vi "20191023_KEK_HEX5.vi"() -> ()   [LabVIEW 2017]
uses:
  <vilib>/DAQmx/create/channels.llb/DAQmx Create Channel (AI-Voltage-Basic).vi
  <vilib>/DAQmx/create/channels.llb/DAQmx Create Channel (AO-Voltage-Basic).vi
  <vilib>/DAQmx/miscellaneous.llb/DAQmx Fill In Error Info.vi
  Lake Shore Cryotronics 218.lvlib
panel:
  out "error D1":errorcluster
  out "error D2":errorcluster
  out "error U3":errorcluster
  out "error D3":errorcluster
  out "error U2":errorcluster
  out "error U1":errorcluster
  out "error S6":errorcluster
  out "error S5":errorcluster
  out "error S4":errorcluster
  out "error S3":errorcluster
  out "error S2":errorcluster
  out "error S1":errorcluster
  in  "Tab Control":T1(tab)
  out "ref LSI-D":refnum<file>
  in  "DAQ IN: P_4HeIN":tag="Dev1/ai16"
  in  "max_P4HeIN":dbl=5.0
  in  "min_P4HeIN":dbl
  in  "DAQ IN: BARA":tag="Dev1/ai7"
  in  "VISA LSI218 DOWN":refnum<visa-resource-name>="GPIB0::11::INSTR"
  in  "DAQ OUT ON?":bool
  out "ref DAQ":refnum<file>
  in  "max_OUT":dbl=5.0
  in  "min_OUT":dbl
  in  "max_FM3":dbl=5.0
  in  "min_FM3":dbl
  in  "max_FM4":dbl=5.0
  in  "min_FM4":dbl
  in  "max_dP3":dbl=5.0
  in  "min_dP3":dbl
  in  "max_dP4":dbl=5.0
  in  "min_dP4":dbl
  in  "max_LM":dbl=0.15
  in  "min_LM":dbl
  in  "max_P":dbl=5.0
  in  "min_P":dbl
  in  "DAQ IN: FM (3He)":tag="Dev1/ai6"
  in  "DAQ IN: FM (4He)":tag="Dev1/ai5"
  in  "DAQ IN: ΔP (3He)":tag="Dev1/ai4"
  in  "DAQ IN: He-level":tag="Dev1/ai2"
  in  "DAQ IN: ΔP (4He)":tag="Dev1/ai3"
  in  "DAQ IN: P (4He coil out)":tag="Dev1/ai1"
  in  "CSV filename suffix":string="TEST_"
  in  "base path":path=path "C:/Users/TUCAN_rcnp/Desktop/Labview/KEK_20191023_HEX5/TEST"
  out "ref LSI-U":refnum<file>
  in  "VISA LSI218 UP":refnum<visa-resource-name>="GPIB0::3::INSTR"
  in  "DAQ OUT":tag="Dev1/ao0"
  in  "sample #":i32=5
  out "error out \n(LSIU)":errorcluster
  out "error out\n(file creation)":errorcluster
  out "error out\n(DAQ config)":errorcluster
  out "error out\n(DAQ OUT)":errorcluster
  out "error out \n(DAQ IN)":errorcluster
  out "error out \n(record LSIU)":errorcluster
  out "error out \n(record DAQ)":errorcluster
  out "error out DAQ Final state":errorcluster
  out "error out \n(LSID)":errorcluster
  in  "max_BARA":dbl=5.0
  in  "min_BARA":dbl
  in  "min_P3HeOUT":dbl
  in  "max_P3HeOUT":dbl=5.0
  in  "DAQ IN: P_3HeOUT":tag="Dev1/ai17"
  out "error out \n(record LSID)":errorcluster
  in  "LSI-D CH":string[](array[string])=["D1", "D2", "D3", "D4", "D5", "D6", "D7", "D8"]
  in  "NI DAQ AIN labels":string[](array[string])=["P_4KRES_COILIN", "LM", "DP_3He", "DP_4He", "FM_4He", "FM_3He", "P_4KRES_BARA", "P_4He_IN", "P_3He_OUT"]
  in  "LSI-U CH labels":string[](array[string])=["U1", "U2", "U3", "U4", "U5", "U6", "U7", "U8"]
  in  "LSI-D CH labels":string[](array[string])=["D1", "D2", "D3", "DISABLED", "D5", "D6", "D7", "D8"]
  in  "LSI-U CH":string[](array[string])=["U1", "U2", "U3", "U4", "U5", "U6", "U7", "U8"]
  in  "DAQ CH":string[](array[string])=["Q1", "Q2", "Q3", "Q4", "Q5", "Q6", "Q7", "Q8", "Q9"]
  out "LSI-U Grpah 1":cluster{dbl[], dbl[]}[](graph)=[{[3644898082.6645026, 3644898087.663789, 3644898092.6640744, 3644898097.66436, 3644898102.6646466, 3644898107.663933, 3644898112.6642184, 3644898117.664504, 3644898122.66379, 3644898127.664076, 3644898132.6643624, 3644898137.665648, 3644898142.6649346, 3644898147.66522, 3644898152.6655064, 3644898157.664792, 3644898162.665078, 3644898167.665364, 3644898172.6656504, 3644898177.664936, 3644898182.665222, 3644898187.665508, 3644898192.6647944, 3644898197.66508, 3644898202.6663666, 3644898207.666652, 3644898212.6659384, 3644898217.666224, 3644898222.6665106, 3644898227.665796, 3644898232.6660824, 3644898237.667368, 3644898242.6676545, 3644898247.66694, 3644898252.6672263, 3644898257.667512, 3644898262.6667986, 3644898267.667084, 3644898272.6673694, 3644898277.667656, 3644898282.6669426, 3644898287.667228, 3644898292.6675134, 3644898297.6678, 3644898302.6680865, 3644898307.668372, 3644898312.668658, 3644898317.667944, 3644898322.6682296, 3644898327.668516, 3644898332.6678014, 3644898337.668088, 3644898342.6683736, 3644898347.66866, 3644898352.6679454, 3644898357.668232, 3644898362.6685176, 3644898367.667804, 3644898372.6680894, 3644898377.668376, 3644898382.6686616, 3644898387.667948, 3644898392.6682334, 3644898397.66852, 3644898402.6678057, 3644898407.6680913, 3644898412.6683774, 3644898417.668664, 3644898422.6679497], [305.66, 305.96, 305.22, 305.33, 305.78, 305.05, 305.43, 306.1, 305.47, 305.83, 305.61, 305.97, 305.69, 305.75, 305.82, 305.82, 305.69, 305.52, 305.52, 306.2, 306.15, 305.92, 305.78, 305.61, 305.73, 305.41, 305.57, 306.24, 306.43, 305.83, 305.97, 306.01, 306.34, 305.78, 305.78, 306.48, 306.2, 306.2, 305.47, 305.96, 305.57, 305.97, 305.83, 305.83, 306.06, 305.92, 305.66, 305.82, 305.64, 305.57, 305.78, 305.73, 306.17, 305.83, 305.9, 306.15, 305.43, 305.87, 306.24, 306.04, 305.82, 306.06, 305.52, 305.75, 306.04, 306.06, 305.48, 305.75, 305.92]}, {[3644898082.6645026, 3644898087.663789, 3644898092.6640744, 3644898097.66436, 3644898102.6646466, 3644898107.663933, 3644898112.6642184, 3644898117.664504, 3644898122.66379, 3644898127.664076, 3644898132.6643624, 3644898137.665648, 3644898142.6649346, 3644898147.66522, 3644898152.6655064, 3644898157.664792, 3644898162.665078, 3644898167.665364, 3644898172.6656504, 3644898177.664936, 3644898182.665222, 3644898187.665508, 3644898192.6647944, 3644898197.66508, 3644898202.6663666, 3644898207.666652, 3644898212.6659384, 3644898217.666224, 3644898222.6665106, 3644898227.665796, 3644898232.6660824, 3644898237.667368, 3644898242.6676545, 3644898247.66694, 3644898252.6672263, 3644898257.667512, 3644898262.6667986, 3644898267.667084, 3644898272.6673694, 3644898277.667656, 3644898282.6669426, 3644898287.667228, 3644898292.6675134, 3644898297.6678, 3644898302.6680865, 3644898307.668372, 3644898312.668658, 3644898317.667944, 3644898322.6682296, 3644898327.668516, 3644898332.6678014, 3644898337.668088, 3644898342.6683736, 3644898347.66866, 3644898352.6679454, 3644898357.668232, 3644898362.6685176, 3644898367.667804, 3644898372.6680894, 3644898377.668376, 3644898382.6686616, 3644898387.667948, 3644898392.6682334, 3644898397.66852, 3644898402.6678057, 3644898407.6680913, 3644898412.6683774, 3644898417.668664, 3644898422.6679497], [296.0, 296.1, 295.89, 295.78, 295.94, 295.91, 295.97, 296.12, 296.01, 296.1, 296.01, 296.2, 296.14, 296.06, 296.16, 296.08, 295.89, 295.97, 296.06, 296.03, 296.09, 295.99, 295.89, 295.85, 295.93, 295.74, 295.91, 296.21, 296.04, 296.14, 296.12, 295.91, 296.2, 295.91, 295.87, 296.09, 296.19, 295.91, 296.03, 296.12, 295.94, 296.03, 295.97, 296.01, 296.08, 295.89, 295.91, 295.97, 296.03, 295.81, 295.91, 296.1, 296.15, 296.05, 296.15, 296.24, 295.82, 295.81, 296.14, 296.24, 295.97, 296.06, 295.74, 295.95, 296.08, 295.94, 295.91, 295.91, 296.12]}, {[3644898082.6645026, 3644898087.663789, 3644898092.6640744, 3644898097.66436, 3644898102.6646466, 3644898107.663933, 3644898112.6642184, 3644898117.664504, 3644898122.66379, 3644898127.664076, 3644898132.6643624, 3644898137.665648, 3644898142.6649346, 3644898147.66522, 3644898152.6655064, 3644898157.664792, 3644898162.665078, 3644898167.665364, 3644898172.6656504, 3644898177.664936, 3644898182.665222, 3644898187.665508, 3644898192.6647944, 3644898197.66508, 3644898202.6663666, 3644898207.666652, 3644898212.6659384, 3644898217.666224, 3644898222.6665106, 3644898227.665796, 3644898232.6660824, 3644898237.667368, 3644898242.6676545, 3644898247.66694, 3644898252.6672263, 3644898257.667512, 3644898262.6667986, 3644898267.667084, 3644898272.6673694, 3644898277.667656, 3644898282.6669426, 3644898287.667228, 3644898292.6675134, 3644898297.6678, 3644898302.6680865, 3644898307.668372, 3644898312.668658, 3644898317.667944, 3644898322.6682296, 3644898327.668516, 3644898332.6678014, 3644898337.668088, 3644898342.6683736, 3644898347.66866, 3644898352.6679454, 3644898357.668232, 3644898362.6685176, 3644898367.667804, 3644898372.6680894, 3644898377.668376, 3644898382.6686616, 3644898387.667948, 3644898392.6682334, 3644898397.66852, 3644898402.6678057, 3644898407.6680913, 3644898412.6683774, 3644898417.668664, 3644898422.6679497], [290.48, 291.09, 290.9, 291.1, 290.9, 290.9, 291.04, 291.04, 290.99, 290.93, 290.9, 291.31, 290.97, 291.13, 291.04, 291.12, 290.93, 290.69, 291.06, 291.27, 291.06, 291.04, 290.96, 291.09, 290.86, 290.95, 291.01, 291.18, 291.25, 291.18, 290.95, 291.08, 291.12, 290.97, 290.93, 291.09, 291.27, 291.02, 290.93, 291.08, 291.22, 291.12, 290.92, 290.69, 291.02, 291.02, 290.9, 290.86, 291.08, 290.88, 290.77, 291.01, 291.05, 291.1, 291.14, 290.99, 291.06, 290.9, 291.05, 291.31, 291.05, 291.06, 290.95, 290.99, 290.99, 290.9, 290.9, 290.96, 291.08]}]
  out "LSI-U CH indic,":string[](array[string])=["U1", "U2", "U3", "U4", "U5", "U6", "U7", "U8"]
  out "LSI-U out":dbl[](array[numeric])=[305.92, 296.12, 291.08, 301.5, 302.08, 302.37, 301.36, 300.38]
  in  "GraphU1 SEL":i32[](array[numeric])=[0, 1]
  out "LSI-D out":dbl[](array[numeric])=[305.92, 296.12, 291.08, 301.5, 302.08, 302.37, 301.36, 300.38]
  out "LSI-D CH indic.":string[](array[string])=["U1", "U2", "U3", "U4", "U5", "U6", "U7", "U8"]
  out "LSI-U Grpah 2":cluster{dbl[], dbl[]}[](graph)=[{[3644898082.6645026, 3644898087.663789, 3644898092.6640744, 3644898097.66436, 3644898102.6646466, 3644898107.663933, 3644898112.6642184, 3644898117.664504, 3644898122.66379, 3644898127.664076, 3644898132.6643624, 3644898137.665648, 3644898142.6649346, 3644898147.66522, 3644898152.6655064, 3644898157.664792, 3644898162.665078, 3644898167.665364, 3644898172.6656504, 3644898177.664936, 3644898182.665222, 3644898187.665508, 3644898192.6647944, 3644898197.66508, 3644898202.6663666, 3644898207.666652, 3644898212.6659384, 3644898217.666224, 3644898222.6665106, 3644898227.665796, 3644898232.6660824, 3644898237.667368, 3644898242.6676545, 3644898247.66694, 3644898252.6672263, 3644898257.667512, 3644898262.6667986, 3644898267.667084, 3644898272.6673694, 3644898277.667656, 3644898282.6669426, 3644898287.667228, 3644898292.6675134, 3644898297.6678, 3644898302.6680865, 3644898307.668372, 3644898312.668658, 3644898317.667944, 3644898322.6682296, 3644898327.668516, 3644898332.6678014, 3644898337.668088, 3644898342.6683736, 3644898347.66866, 3644898352.6679454, 3644898357.668232, 3644898362.6685176, 3644898367.667804, 3644898372.6680894, 3644898377.668376, 3644898382.6686616, 3644898387.667948, 3644898392.6682334, 3644898397.66852, 3644898402.6678057, 3644898407.6680913, 3644898412.6683774, 3644898417.668664, 3644898422.6679497], [305.66, 305.96, 305.22, 305.33, 305.78, 305.05, 305.43, 306.1, 305.47, 305.83, 305.61, 305.97, 305.69, 305.75, 305.82, 305.82, 305.69, 305.52, 305.52, 306.2, 306.15, 305.92, 305.78, 305.61, 305.73, 305.41, 305.57, 306.24, 306.43, 305.83, 305.97, 306.01, 306.34, 305.78, 305.78, 306.48, 306.2, 306.2, 305.47, 305.96, 305.57, 305.97, 305.83, 305.83, 306.06, 305.92, 305.66, 305.82, 305.64, 305.57, 305.78, 305.73, 306.17, 305.83, 305.9, 306.15, 305.43, 305.87, 306.24, 306.04, 305.82, 306.06, 305.52, 305.75, 306.04, 306.06, 305.48, 305.75, 305.92]}, {[3644898082.6645026, 3644898087.663789, 3644898092.6640744, 3644898097.66436, 3644898102.6646466, 3644898107.663933, 3644898112.6642184, 3644898117.664504, 3644898122.66379, 3644898127.664076, 3644898132.6643624, 3644898137.665648, 3644898142.6649346, 3644898147.66522, 3644898152.6655064, 3644898157.664792, 3644898162.665078, 3644898167.665364, 3644898172.6656504, 3644898177.664936, 3644898182.665222, 3644898187.665508, 3644898192.6647944, 3644898197.66508, 3644898202.6663666, 3644898207.666652, 3644898212.6659384, 3644898217.666224, 3644898222.6665106, 3644898227.665796, 3644898232.6660824, 3644898237.667368, 3644898242.6676545, 3644898247.66694, 3644898252.6672263, 3644898257.667512, 3644898262.6667986, 3644898267.667084, 3644898272.6673694, 3644898277.667656, 3644898282.6669426, 3644898287.667228, 3644898292.6675134, 3644898297.6678, 3644898302.6680865, 3644898307.668372, 3644898312.668658, 3644898317.667944, 3644898322.6682296, 3644898327.668516, 3644898332.6678014, 3644898337.668088, 3644898342.6683736, 3644898347.66866, 3644898352.6679454, 3644898357.668232, 3644898362.6685176, 3644898367.667804, 3644898372.6680894, 3644898377.668376, 3644898382.6686616, 3644898387.667948, 3644898392.6682334, 3644898397.66852, 3644898402.6678057, 3644898407.6680913, 3644898412.6683774, 3644898417.668664, 3644898422.6679497], [296.0, 296.1, 295.89, 295.78, 295.94, 295.91, 295.97, 296.12, 296.01, 296.1, 296.01, 296.2, 296.14, 296.06, 296.16, 296.08, 295.89, 295.97, 296.06, 296.03, 296.09, 295.99, 295.89, 295.85, 295.93, 295.74, 295.91, 296.21, 296.04, 296.14, 296.12, 295.91, 296.2, 295.91, 295.87, 296.09, 296.19, 295.91, 296.03, 296.12, 295.94, 296.03, 295.97, 296.01, 296.08, 295.89, 295.91, 295.97, 296.03, 295.81, 295.91, 296.1, 296.15, 296.05, 296.15, 296.24, 295.82, 295.81, 296.14, 296.24, 295.97, 296.06, 295.74, 295.95, 296.08, 295.94, 295.91, 295.91, 296.12]}, {[3644898082.6645026, 3644898087.663789, 3644898092.6640744, 3644898097.66436, 3644898102.6646466, 3644898107.663933, 3644898112.6642184, 3644898117.664504, 3644898122.66379, 3644898127.664076, 3644898132.6643624, 3644898137.665648, 3644898142.6649346, 3644898147.66522, 3644898152.6655064, 3644898157.664792, 3644898162.665078, 3644898167.665364, 3644898172.6656504, 3644898177.664936, 3644898182.665222, 3644898187.665508, 3644898192.6647944, 3644898197.66508, 3644898202.6663666, 3644898207.666652, 3644898212.6659384, 3644898217.666224, 3644898222.6665106, 3644898227.665796, 3644898232.6660824, 3644898237.667368, 3644898242.6676545, 3644898247.66694, 3644898252.6672263, 3644898257.667512, 3644898262.6667986, 3644898267.667084, 3644898272.6673694, 3644898277.667656, 3644898282.6669426, 3644898287.667228, 3644898292.6675134, 3644898297.6678, 3644898302.6680865, 3644898307.668372, 3644898312.668658, 3644898317.667944, 3644898322.6682296, 3644898327.668516, 3644898332.6678014, 3644898337.668088, 3644898342.6683736, 3644898347.66866, 3644898352.6679454, 3644898357.668232, 3644898362.6685176, 3644898367.667804, 3644898372.6680894, 3644898377.668376, 3644898382.6686616, 3644898387.667948, 3644898392.6682334, 3644898397.66852, 3644898402.6678057, 3644898407.6680913, 3644898412.6683774, 3644898417.668664, 3644898422.6679497], [290.48, 291.09, 290.9, 291.1, 290.9, 290.9, 291.04, 291.04, 290.99, 290.93, 290.9, 291.31, 290.97, 291.13, 291.04, 291.12, 290.93, 290.69, 291.06, 291.27, 291.06, 291.04, 290.96, 291.09, 290.86, 290.95, 291.01, 291.18, 291.25, 291.18, 290.95, 291.08, 291.12, 290.97, 290.93, 291.09, 291.27, 291.02, 290.93, 291.08, 291.22, 291.12, 290.92, 290.69, 291.02, 291.02, 290.9, 290.86, 291.08, 290.88, 290.77, 291.01, 291.05, 291.1, 291.14, 290.99, 291.06, 290.9, 291.05, 291.31, 291.05, 291.06, 290.95, 290.99, 290.99, 290.9, 290.9, 290.96, 291.08]}]
  in  "GraphU2 SEL":i32[](array[numeric])=[2, 3, 4]
  in  "GraphU3 SEL":i32[](array[numeric])=[5, 6, 6]
  out "LSI-U Grpah 3":cluster{dbl[], dbl[]}[](graph)=[{[3644898082.6645026, 3644898087.663789, 3644898092.6640744, 3644898097.66436, 3644898102.6646466, 3644898107.663933, 3644898112.6642184, 3644898117.664504, 3644898122.66379, 3644898127.664076, 3644898132.6643624, 3644898137.665648, 3644898142.6649346, 3644898147.66522, 3644898152.6655064, 3644898157.664792, 3644898162.665078, 3644898167.665364, 3644898172.6656504, 3644898177.664936, 3644898182.665222, 3644898187.665508, 3644898192.6647944, 3644898197.66508, 3644898202.6663666, 3644898207.666652, 3644898212.6659384, 3644898217.666224, 3644898222.6665106, 3644898227.665796, 3644898232.6660824, 3644898237.667368, 3644898242.6676545, 3644898247.66694, 3644898252.6672263, 3644898257.667512, 3644898262.6667986, 3644898267.667084, 3644898272.6673694, 3644898277.667656, 3644898282.6669426, 3644898287.667228, 3644898292.6675134, 3644898297.6678, 3644898302.6680865, 3644898307.668372, 3644898312.668658, 3644898317.667944, 3644898322.6682296, 3644898327.668516, 3644898332.6678014, 3644898337.668088, 3644898342.6683736, 3644898347.66866, 3644898352.6679454, 3644898357.668232, 3644898362.6685176, 3644898367.667804, 3644898372.6680894, 3644898377.668376, 3644898382.6686616, 3644898387.667948, 3644898392.6682334, 3644898397.66852, 3644898402.6678057, 3644898407.6680913, 3644898412.6683774, 3644898417.668664, 3644898422.6679497], [305.66, 305.96, 305.22, 305.33, 305.78, 305.05, 305.43, 306.1, 305.47, 305.83, 305.61, 305.97, 305.69, 305.75, 305.82, 305.82, 305.69, 305.52, 305.52, 306.2, 306.15, 305.92, 305.78, 305.61, 305.73, 305.41, 305.57, 306.24, 306.43, 305.83, 305.97, 306.01, 306.34, 305.78, 305.78, 306.48, 306.2, 306.2, 305.47, 305.96, 305.57, 305.97, 305.83, 305.83, 306.06, 305.92, 305.66, 305.82, 305.64, 305.57, 305.78, 305.73, 306.17, 305.83, 305.9, 306.15, 305.43, 305.87, 306.24, 306.04, 305.82, 306.06, 305.52, 305.75, 306.04, 306.06, 305.48, 305.75, 305.92]}, {[3644898082.6645026, 3644898087.663789, 3644898092.6640744, 3644898097.66436, 3644898102.6646466, 3644898107.663933, 3644898112.6642184, 3644898117.664504, 3644898122.66379, 3644898127.664076, 3644898132.6643624, 3644898137.665648, 3644898142.6649346, 3644898147.66522, 3644898152.6655064, 3644898157.664792, 3644898162.665078, 3644898167.665364, 3644898172.6656504, 3644898177.664936, 3644898182.665222, 3644898187.665508, 3644898192.6647944, 3644898197.66508, 3644898202.6663666, 3644898207.666652, 3644898212.6659384, 3644898217.666224, 3644898222.6665106, 3644898227.665796, 3644898232.6660824, 3644898237.667368, 3644898242.6676545, 3644898247.66694, 3644898252.6672263, 3644898257.667512, 3644898262.6667986, 3644898267.667084, 3644898272.6673694, 3644898277.667656, 3644898282.6669426, 3644898287.667228, 3644898292.6675134, 3644898297.6678, 3644898302.6680865, 3644898307.668372, 3644898312.668658, 3644898317.667944, 3644898322.6682296, 3644898327.668516, 3644898332.6678014, 3644898337.668088, 3644898342.6683736, 3644898347.66866, 3644898352.6679454, 3644898357.668232, 3644898362.6685176, 3644898367.667804, 3644898372.6680894, 3644898377.668376, 3644898382.6686616, 3644898387.667948, 3644898392.6682334, 3644898397.66852, 3644898402.6678057, 3644898407.6680913, 3644898412.6683774, 3644898417.668664, 3644898422.6679497], [296.0, 296.1, 295.89, 295.78, 295.94, 295.91, 295.97, 296.12, 296.01, 296.1, 296.01, 296.2, 296.14, 296.06, 296.16, 296.08, 295.89, 295.97, 296.06, 296.03, 296.09, 295.99, 295.89, 295.85, 295.93, 295.74, 295.91, 296.21, 296.04, 296.14, 296.12, 295.91, 296.2, 295.91, 295.87, 296.09, 296.19, 295.91, 296.03, 296.12, 295.94, 296.03, 295.97, 296.01, 296.08, 295.89, 295.91, 295.97, 296.03, 295.81, 295.91, 296.1, 296.15, 296.05, 296.15, 296.24, 295.82, 295.81, 296.14, 296.24, 295.97, 296.06, 295.74, 295.95, 296.08, 295.94, 295.91, 295.91, 296.12]}, {[3644898082.6645026, 3644898087.663789, 3644898092.6640744, 3644898097.66436, 3644898102.6646466, 3644898107.663933, 3644898112.6642184, 3644898117.664504, 3644898122.66379, 3644898127.664076, 3644898132.6643624, 3644898137.665648, 3644898142.6649346, 3644898147.66522, 3644898152.6655064, 3644898157.664792, 3644898162.665078, 3644898167.665364, 3644898172.6656504, 3644898177.664936, 3644898182.665222, 3644898187.665508, 3644898192.6647944, 3644898197.66508, 3644898202.6663666, 3644898207.666652, 3644898212.6659384, 3644898217.666224, 3644898222.6665106, 3644898227.665796, 3644898232.6660824, 3644898237.667368, 3644898242.6676545, 3644898247.66694, 3644898252.6672263, 3644898257.667512, 3644898262.6667986, 3644898267.667084, 3644898272.6673694, 3644898277.667656, 3644898282.6669426, 3644898287.667228, 3644898292.6675134, 3644898297.6678, 3644898302.6680865, 3644898307.668372, 3644898312.668658, 3644898317.667944, 3644898322.6682296, 3644898327.668516, 3644898332.6678014, 3644898337.668088, 3644898342.6683736, 3644898347.66866, 3644898352.6679454, 3644898357.668232, 3644898362.6685176, 3644898367.667804, 3644898372.6680894, 3644898377.668376, 3644898382.6686616, 3644898387.667948, 3644898392.6682334, 3644898397.66852, 3644898402.6678057, 3644898407.6680913, 3644898412.6683774, 3644898417.668664, 3644898422.6679497], [290.48, 291.09, 290.9, 291.1, 290.9, 290.9, 291.04, 291.04, 290.99, 290.93, 290.9, 291.31, 290.97, 291.13, 291.04, 291.12, 290.93, 290.69, 291.06, 291.27, 291.06, 291.04, 290.96, 291.09, 290.86, 290.95, 291.01, 291.18, 291.25, 291.18, 290.95, 291.08, 291.12, 290.97, 290.93, 291.09, 291.27, 291.02, 290.93, 291.08, 291.22, 291.12, 290.92, 290.69, 291.02, 291.02, 290.9, 290.86, 291.08, 290.88, 290.77, 291.01, 291.05, 291.1, 291.14, 290.99, 291.06, 290.9, 291.05, 291.31, 291.05, 291.06, 290.95, 290.99, 290.99, 290.9, 290.9, 290.96, 291.08]}]
  out "LSI-D Grpah 2":cluster{dbl[], dbl[]}[](graph)=[{[3644898082.6645026, 3644898087.663789, 3644898092.6640744, 3644898097.66436, 3644898102.6646466, 3644898107.663933, 3644898112.6642184, 3644898117.664504, 3644898122.66379, 3644898127.664076, 3644898132.6643624, 3644898137.665648, 3644898142.6649346, 3644898147.66522, 3644898152.6655064, 3644898157.664792, 3644898162.665078, 3644898167.665364, 3644898172.6656504, 3644898177.664936, 3644898182.665222, 3644898187.665508, 3644898192.6647944, 3644898197.66508, 3644898202.6663666, 3644898207.666652, 3644898212.6659384, 3644898217.666224, 3644898222.6665106, 3644898227.665796, 3644898232.6660824, 3644898237.667368, 3644898242.6676545, 3644898247.66694, 3644898252.6672263, 3644898257.667512, 3644898262.6667986, 3644898267.667084, 3644898272.6673694, 3644898277.667656, 3644898282.6669426, 3644898287.667228, 3644898292.6675134, 3644898297.6678, 3644898302.6680865, 3644898307.668372, 3644898312.668658, 3644898317.667944, 3644898322.6682296, 3644898327.668516, 3644898332.6678014, 3644898337.668088, 3644898342.6683736, 3644898347.66866, 3644898352.6679454, 3644898357.668232, 3644898362.6685176, 3644898367.667804, 3644898372.6680894, 3644898377.668376, 3644898382.6686616, 3644898387.667948, 3644898392.6682334, 3644898397.66852, 3644898402.6678057, 3644898407.6680913, 3644898412.6683774, 3644898417.668664, 3644898422.6679497], [305.66, 305.96, 305.22, 305.33, 305.78, 305.05, 305.43, 306.1, 305.47, 305.83, 305.61, 305.97, 305.69, 305.75, 305.82, 305.82, 305.69, 305.52, 305.52, 306.2, 306.15, 305.92, 305.78, 305.61, 305.73, 305.41, 305.57, 306.24, 306.43, 305.83, 305.97, 306.01, 306.34, 305.78, 305.78, 306.48, 306.2, 306.2, 305.47, 305.96, 305.57, 305.97, 305.83, 305.83, 306.06, 305.92, 305.66, 305.82, 305.64, 305.57, 305.78, 305.73, 306.17, 305.83, 305.9, 306.15, 305.43, 305.87, 306.24, 306.04, 305.82, 306.06, 305.52, 305.75, 306.04, 306.06, 305.48, 305.75, 305.92]}, {[3644898082.6645026, 3644898087.663789, 3644898092.6640744, 3644898097.66436, 3644898102.6646466, 3644898107.663933, 3644898112.6642184, 3644898117.664504, 3644898122.66379, 3644898127.664076, 3644898132.6643624, 3644898137.665648, 3644898142.6649346, 3644898147.66522, 3644898152.6655064, 3644898157.664792, 3644898162.665078, 3644898167.665364, 3644898172.6656504, 3644898177.664936, 3644898182.665222, 3644898187.665508, 3644898192.6647944, 3644898197.66508, 3644898202.6663666, 3644898207.666652, 3644898212.6659384, 3644898217.666224, 3644898222.6665106, 3644898227.665796, 3644898232.6660824, 3644898237.667368, 3644898242.6676545, 3644898247.66694, 3644898252.6672263, 3644898257.667512, 3644898262.6667986, 3644898267.667084, 3644898272.6673694, 3644898277.667656, 3644898282.6669426, 3644898287.667228, 3644898292.6675134, 3644898297.6678, 3644898302.6680865, 3644898307.668372, 3644898312.668658, 3644898317.667944, 3644898322.6682296, 3644898327.668516, 3644898332.6678014, 3644898337.668088, 3644898342.6683736, 3644898347.66866, 3644898352.6679454, 3644898357.668232, 3644898362.6685176, 3644898367.667804, 3644898372.6680894, 3644898377.668376, 3644898382.6686616, 3644898387.667948, 3644898392.6682334, 3644898397.66852, 3644898402.6678057, 3644898407.6680913, 3644898412.6683774, 3644898417.668664, 3644898422.6679497], [296.0, 296.1, 295.89, 295.78, 295.94, 295.91, 295.97, 296.12, 296.01, 296.1, 296.01, 296.2, 296.14, 296.06, 296.16, 296.08, 295.89, 295.97, 296.06, 296.03, 296.09, 295.99, 295.89, 295.85, 295.93, 295.74, 295.91, 296.21, 296.04, 296.14, 296.12, 295.91, 296.2, 295.91, 295.87, 296.09, 296.19, 295.91, 296.03, 296.12, 295.94, 296.03, 295.97, 296.01, 296.08, 295.89, 295.91, 295.97, 296.03, 295.81, 295.91, 296.1, 296.15, 296.05, 296.15, 296.24, 295.82, 295.81, 296.14, 296.24, 295.97, 296.06, 295.74, 295.95, 296.08, 295.94, 295.91, 295.91, 296.12]}, {[3644898082.6645026, 3644898087.663789, 3644898092.6640744, 3644898097.66436, 3644898102.6646466, 3644898107.663933, 3644898112.6642184, 3644898117.664504, 3644898122.66379, 3644898127.664076, 3644898132.6643624, 3644898137.665648, 3644898142.6649346, 3644898147.66522, 3644898152.6655064, 3644898157.664792, 3644898162.665078, 3644898167.665364, 3644898172.6656504, 3644898177.664936, 3644898182.665222, 3644898187.665508, 3644898192.6647944, 3644898197.66508, 3644898202.6663666, 3644898207.666652, 3644898212.6659384, 3644898217.666224, 3644898222.6665106, 3644898227.665796, 3644898232.6660824, 3644898237.667368, 3644898242.6676545, 3644898247.66694, 3644898252.6672263, 3644898257.667512, 3644898262.6667986, 3644898267.667084, 3644898272.6673694, 3644898277.667656, 3644898282.6669426, 3644898287.667228, 3644898292.6675134, 3644898297.6678, 3644898302.6680865, 3644898307.668372, 3644898312.668658, 3644898317.667944, 3644898322.6682296, 3644898327.668516, 3644898332.6678014, 3644898337.668088, 3644898342.6683736, 3644898347.66866, 3644898352.6679454, 3644898357.668232, 3644898362.6685176, 3644898367.667804, 3644898372.6680894, 3644898377.668376, 3644898382.6686616, 3644898387.667948, 3644898392.6682334, 3644898397.66852, 3644898402.6678057, 3644898407.6680913, 3644898412.6683774, 3644898417.668664, 3644898422.6679497], [290.48, 291.09, 290.9, 291.1, 290.9, 290.9, 291.04, 291.04, 290.99, 290.93, 290.9, 291.31, 290.97, 291.13, 291.04, 291.12, 290.93, 290.69, 291.06, 291.27, 291.06, 291.04, 290.96, 291.09, 290.86, 290.95, 291.01, 291.18, 291.25, 291.18, 290.95, 291.08, 291.12, 290.97, 290.93, 291.09, 291.27, 291.02, 290.93, 291.08, 291.22, 291.12, 290.92, 290.69, 291.02, 291.02, 290.9, 290.86, 291.08, 290.88, 290.77, 291.01, 291.05, 291.1, 291.14, 290.99, 291.06, 290.9, 291.05, 291.31, 291.05, 291.06, 290.95, 290.99, 290.99, 290.9, 290.9, 290.96, 291.08]}]
  out "LSI-D Grpah 3":cluster{dbl[], dbl[]}[](graph)=[{[3644898082.6645026, 3644898087.663789, 3644898092.6640744, 3644898097.66436, 3644898102.6646466, 3644898107.663933, 3644898112.6642184, 3644898117.664504, 3644898122.66379, 3644898127.664076, 3644898132.6643624, 3644898137.665648, 3644898142.6649346, 3644898147.66522, 3644898152.6655064, 3644898157.664792, 3644898162.665078, 3644898167.665364, 3644898172.6656504, 3644898177.664936, 3644898182.665222, 3644898187.665508, 3644898192.6647944, 3644898197.66508, 3644898202.6663666, 3644898207.666652, 3644898212.6659384, 3644898217.666224, 3644898222.6665106, 3644898227.665796, 3644898232.6660824, 3644898237.667368, 3644898242.6676545, 3644898247.66694, 3644898252.6672263, 3644898257.667512, 3644898262.6667986, 3644898267.667084, 3644898272.6673694, 3644898277.667656, 3644898282.6669426, 3644898287.667228, 3644898292.6675134, 3644898297.6678, 3644898302.6680865, 3644898307.668372, 3644898312.668658, 3644898317.667944, 3644898322.6682296, 3644898327.668516, 3644898332.6678014, 3644898337.668088, 3644898342.6683736, 3644898347.66866, 3644898352.6679454, 3644898357.668232, 3644898362.6685176, 3644898367.667804, 3644898372.6680894, 3644898377.668376, 3644898382.6686616, 3644898387.667948, 3644898392.6682334, 3644898397.66852, 3644898402.6678057, 3644898407.6680913, 3644898412.6683774, 3644898417.668664, 3644898422.6679497], [305.66, 305.96, 305.22, 305.33, 305.78, 305.05, 305.43, 306.1, 305.47, 305.83, 305.61, 305.97, 305.69, 305.75, 305.82, 305.82, 305.69, 305.52, 305.52, 306.2, 306.15, 305.92, 305.78, 305.61, 305.73, 305.41, 305.57, 306.24, 306.43, 305.83, 305.97, 306.01, 306.34, 305.78, 305.78, 306.48, 306.2, 306.2, 305.47, 305.96, 305.57, 305.97, 305.83, 305.83, 306.06, 305.92, 305.66, 305.82, 305.64, 305.57, 305.78, 305.73, 306.17, 305.83, 305.9, 306.15, 305.43, 305.87, 306.24, 306.04, 305.82, 306.06, 305.52, 305.75, 306.04, 306.06, 305.48, 305.75, 305.92]}, {[3644898082.6645026, 3644898087.663789, 3644898092.6640744, 3644898097.66436, 3644898102.6646466, 3644898107.663933, 3644898112.6642184, 3644898117.664504, 3644898122.66379, 3644898127.664076, 3644898132.6643624, 3644898137.665648, 3644898142.6649346, 3644898147.66522, 3644898152.6655064, 3644898157.664792, 3644898162.665078, 3644898167.665364, 3644898172.6656504, 3644898177.664936, 3644898182.665222, 3644898187.665508, 3644898192.6647944, 3644898197.66508, 3644898202.6663666, 3644898207.666652, 3644898212.6659384, 3644898217.666224, 3644898222.6665106, 3644898227.665796, 3644898232.6660824, 3644898237.667368, 3644898242.6676545, 3644898247.66694, 3644898252.6672263, 3644898257.667512, 3644898262.6667986, 3644898267.667084, 3644898272.6673694, 3644898277.667656, 3644898282.6669426, 3644898287.667228, 3644898292.6675134, 3644898297.6678, 3644898302.6680865, 3644898307.668372, 3644898312.668658, 3644898317.667944, 3644898322.6682296, 3644898327.668516, 3644898332.6678014, 3644898337.668088, 3644898342.6683736, 3644898347.66866, 3644898352.6679454, 3644898357.668232, 3644898362.6685176, 3644898367.667804, 3644898372.6680894, 3644898377.668376, 3644898382.6686616, 3644898387.667948, 3644898392.6682334, 3644898397.66852, 3644898402.6678057, 3644898407.6680913, 3644898412.6683774, 3644898417.668664, 3644898422.6679497], [296.0, 296.1, 295.89, 295.78, 295.94, 295.91, 295.97, 296.12, 296.01, 296.1, 296.01, 296.2, 296.14, 296.06, 296.16, 296.08, 295.89, 295.97, 296.06, 296.03, 296.09, 295.99, 295.89, 295.85, 295.93, 295.74, 295.91, 296.21, 296.04, 296.14, 296.12, 295.91, 296.2, 295.91, 295.87, 296.09, 296.19, 295.91, 296.03, 296.12, 295.94, 296.03, 295.97, 296.01, 296.08, 295.89, 295.91, 295.97, 296.03, 295.81, 295.91, 296.1, 296.15, 296.05, 296.15, 296.24, 295.82, 295.81, 296.14, 296.24, 295.97, 296.06, 295.74, 295.95, 296.08, 295.94, 295.91, 295.91, 296.12]}, {[3644898082.6645026, 3644898087.663789, 3644898092.6640744, 3644898097.66436, 3644898102.6646466, 3644898107.663933, 3644898112.6642184, 3644898117.664504, 3644898122.66379, 3644898127.664076, 3644898132.6643624, 3644898137.665648, 3644898142.6649346, 3644898147.66522, 3644898152.6655064, 3644898157.664792, 3644898162.665078, 3644898167.665364, 3644898172.6656504, 3644898177.664936, 3644898182.665222, 3644898187.665508, 3644898192.6647944, 3644898197.66508, 3644898202.6663666, 3644898207.666652, 3644898212.6659384, 3644898217.666224, 3644898222.6665106, 3644898227.665796, 3644898232.6660824, 3644898237.667368, 3644898242.6676545, 3644898247.66694, 3644898252.6672263, 3644898257.667512, 3644898262.6667986, 3644898267.667084, 3644898272.6673694, 3644898277.667656, 3644898282.6669426, 3644898287.667228, 3644898292.6675134, 3644898297.6678, 3644898302.6680865, 3644898307.668372, 3644898312.668658, 3644898317.667944, 3644898322.6682296, 3644898327.668516, 3644898332.6678014, 3644898337.668088, 3644898342.6683736, 3644898347.66866, 3644898352.6679454, 3644898357.668232, 3644898362.6685176, 3644898367.667804, 3644898372.6680894, 3644898377.668376, 3644898382.6686616, 3644898387.667948, 3644898392.6682334, 3644898397.66852, 3644898402.6678057, 3644898407.6680913, 3644898412.6683774, 3644898417.668664, 3644898422.6679497], [290.48, 291.09, 290.9, 291.1, 290.9, 290.9, 291.04, 291.04, 290.99, 290.93, 290.9, 291.31, 290.97, 291.13, 291.04, 291.12, 290.93, 290.69, 291.06, 291.27, 291.06, 291.04, 290.96, 291.09, 290.86, 290.95, 291.01, 291.18, 291.25, 291.18, 290.95, 291.08, 291.12, 290.97, 290.93, 291.09, 291.27, 291.02, 290.93, 291.08, 291.22, 291.12, 290.92, 290.69, 291.02, 291.02, 290.9, 290.86, 291.08, 290.88, 290.77, 291.01, 291.05, 291.1, 291.14, 290.99, 291.06, 290.9, 291.05, 291.31, 291.05, 291.06, 290.95, 290.99, 290.99, 290.9, 290.9, 290.96, 291.08]}]
  in  "GraphD1 SEL":i32[](array[numeric])=[0, 1]
  out "LSI-D Grpah 1":cluster{dbl[], dbl[]}[](graph)=[{[3644898082.6645026, 3644898087.663789, 3644898092.6640744, 3644898097.66436, 3644898102.6646466, 3644898107.663933, 3644898112.6642184, 3644898117.664504, 3644898122.66379, 3644898127.664076, 3644898132.6643624, 3644898137.665648, 3644898142.6649346, 3644898147.66522, 3644898152.6655064, 3644898157.664792, 3644898162.665078, 3644898167.665364, 3644898172.6656504, 3644898177.664936, 3644898182.665222, 3644898187.665508, 3644898192.6647944, 3644898197.66508, 3644898202.6663666, 3644898207.666652, 3644898212.6659384, 3644898217.666224, 3644898222.6665106, 3644898227.665796, 3644898232.6660824, 3644898237.667368, 3644898242.6676545, 3644898247.66694, 3644898252.6672263, 3644898257.667512, 3644898262.6667986, 3644898267.667084, 3644898272.6673694, 3644898277.667656, 3644898282.6669426, 3644898287.667228, 3644898292.6675134, 3644898297.6678, 3644898302.6680865, 3644898307.668372, 3644898312.668658, 3644898317.667944, 3644898322.6682296, 3644898327.668516, 3644898332.6678014, 3644898337.668088, 3644898342.6683736, 3644898347.66866, 3644898352.6679454, 3644898357.668232, 3644898362.6685176, 3644898367.667804, 3644898372.6680894, 3644898377.668376, 3644898382.6686616, 3644898387.667948, 3644898392.6682334, 3644898397.66852, 3644898402.6678057, 3644898407.6680913, 3644898412.6683774, 3644898417.668664, 3644898422.6679497], [305.66, 305.96, 305.22, 305.33, 305.78, 305.05, 305.43, 306.1, 305.47, 305.83, 305.61, 305.97, 305.69, 305.75, 305.82, 305.82, 305.69, 305.52, 305.52, 306.2, 306.15, 305.92, 305.78, 305.61, 305.73, 305.41, 305.57, 306.24, 306.43, 305.83, 305.97, 306.01, 306.34, 305.78, 305.78, 306.48, 306.2, 306.2, 305.47, 305.96, 305.57, 305.97, 305.83, 305.83, 306.06, 305.92, 305.66, 305.82, 305.64, 305.57, 305.78, 305.73, 306.17, 305.83, 305.9, 306.15, 305.43, 305.87, 306.24, 306.04, 305.82, 306.06, 305.52, 305.75, 306.04, 306.06, 305.48, 305.75, 305.92]}, {[3644898082.6645026, 3644898087.663789, 3644898092.6640744, 3644898097.66436, 3644898102.6646466, 3644898107.663933, 3644898112.6642184, 3644898117.664504, 3644898122.66379, 3644898127.664076, 3644898132.6643624, 3644898137.665648, 3644898142.6649346, 3644898147.66522, 3644898152.6655064, 3644898157.664792, 3644898162.665078, 3644898167.665364, 3644898172.6656504, 3644898177.664936, 3644898182.665222, 3644898187.665508, 3644898192.6647944, 3644898197.66508, 3644898202.6663666, 3644898207.666652, 3644898212.6659384, 3644898217.666224, 3644898222.6665106, 3644898227.665796, 3644898232.6660824, 3644898237.667368, 3644898242.6676545, 3644898247.66694, 3644898252.6672263, 3644898257.667512, 3644898262.6667986, 3644898267.667084, 3644898272.6673694, 3644898277.667656, 3644898282.6669426, 3644898287.667228, 3644898292.6675134, 3644898297.6678, 3644898302.6680865, 3644898307.668372, 3644898312.668658, 3644898317.667944, 3644898322.6682296, 3644898327.668516, 3644898332.6678014, 3644898337.668088, 3644898342.6683736, 3644898347.66866, 3644898352.6679454, 3644898357.668232, 3644898362.6685176, 3644898367.667804, 3644898372.6680894, 3644898377.668376, 3644898382.6686616, 3644898387.667948, 3644898392.6682334, 3644898397.66852, 3644898402.6678057, 3644898407.6680913, 3644898412.6683774, 3644898417.668664, 3644898422.6679497], [296.0, 296.1, 295.89, 295.78, 295.94, 295.91, 295.97, 296.12, 296.01, 296.1, 296.01, 296.2, 296.14, 296.06, 296.16, 296.08, 295.89, 295.97, 296.06, 296.03, 296.09, 295.99, 295.89, 295.85, 295.93, 295.74, 295.91, 296.21, 296.04, 296.14, 296.12, 295.91, 296.2, 295.91, 295.87, 296.09, 296.19, 295.91, 296.03, 296.12, 295.94, 296.03, 295.97, 296.01, 296.08, 295.89, 295.91, 295.97, 296.03, 295.81, 295.91, 296.1, 296.15, 296.05, 296.15, 296.24, 295.82, 295.81, 296.14, 296.24, 295.97, 296.06, 295.74, 295.95, 296.08, 295.94, 295.91, 295.91, 296.12]}, {[3644898082.6645026, 3644898087.663789, 3644898092.6640744, 3644898097.66436, 3644898102.6646466, 3644898107.663933, 3644898112.6642184, 3644898117.664504, 3644898122.66379, 3644898127.664076, 3644898132.6643624, 3644898137.665648, 3644898142.6649346, 3644898147.66522, 3644898152.6655064, 3644898157.664792, 3644898162.665078, 3644898167.665364, 3644898172.6656504, 3644898177.664936, 3644898182.665222, 3644898187.665508, 3644898192.6647944, 3644898197.66508, 3644898202.6663666, 3644898207.666652, 3644898212.6659384, 3644898217.666224, 3644898222.6665106, 3644898227.665796, 3644898232.6660824, 3644898237.667368, 3644898242.6676545, 3644898247.66694, 3644898252.6672263, 3644898257.667512, 3644898262.6667986, 3644898267.667084, 3644898272.6673694, 3644898277.667656, 3644898282.6669426, 3644898287.667228, 3644898292.6675134, 3644898297.6678, 3644898302.6680865, 3644898307.668372, 3644898312.668658, 3644898317.667944, 3644898322.6682296, 3644898327.668516, 3644898332.6678014, 3644898337.668088, 3644898342.6683736, 3644898347.66866, 3644898352.6679454, 3644898357.668232, 3644898362.6685176, 3644898367.667804, 3644898372.6680894, 3644898377.668376, 3644898382.6686616, 3644898387.667948, 3644898392.6682334, 3644898397.66852, 3644898402.6678057, 3644898407.6680913, 3644898412.6683774, 3644898417.668664, 3644898422.6679497], [290.48, 291.09, 290.9, 291.1, 290.9, 290.9, 291.04, 291.04, 290.99, 290.93, 290.9, 291.31, 290.97, 291.13, 291.04, 291.12, 290.93, 290.69, 291.06, 291.27, 291.06, 291.04, 290.96, 291.09, 290.86, 290.95, 291.01, 291.18, 291.25, 291.18, 290.95, 291.08, 291.12, 290.97, 290.93, 291.09, 291.27, 291.02, 290.93, 291.08, 291.22, 291.12, 290.92, 290.69, 291.02, 291.02, 290.9, 290.86, 291.08, 290.88, 290.77, 291.01, 291.05, 291.1, 291.14, 290.99, 291.06, 290.9, 291.05, 291.31, 291.05, 291.06, 290.95, 290.99, 290.99, 290.9, 290.9, 290.96, 291.08]}]
  in  "GraphD2 SEL":i32[](array[numeric])=[2, 3, 4]
  in  "GraphD3 SEL":i32[](array[numeric])=[5, 6, 6]
  out "Graph S. 6":cluster{dbl[], dbl[]}[](graph)
  in  "S.6 SEL":i32[](array[numeric])=[0, 2, 3]
  in  "log/linear 6":bool
  in  "log/linear 5":bool
  in  "S.5 SEL":i32[](array[numeric])=[0, 2, 3]
  in  "log/linear 4":bool
  in  "S.4 SEL":i32[](array[numeric])=[0, 2, 3]
  in  "log/linear 3":bool
  in  "log/linear 1":bool
  in  "unit":string[](array[string])=["Pa", "%", "Pa", "Pa", "L/min", "L/min", "Pa", "Pa", "Pa"]
  out "NI DAQ OUT":dbl[](array[numeric])=[-50013.24569663551, 15.025355709698363, -250.03334959533717, -250.04156931728906, -26.29672579614668, -0.7155199244462975, 103537.91205606361, -50000.0, -50000.0] format="%#_3f"
  out "NI-DAQ CH indic.":string[](array[string])=["U1", "U2", "U3", "U4", "U5", "U6", "U7", "U8"]
  out "Graph S. 1":cluster{dbl[], dbl[]}[](graph)
  in  "S.1 SEL":i32[](array[numeric])=[0, 2]
  out "Graph S. 2":cluster{dbl[], dbl[]}[](graph)
  in  "S.2 SEL":i32[](array[numeric])=[1]
  in  "log/linear 2":bool
  out "Graph S. 3":cluster{dbl[], dbl[]}[](graph)
  in  "S.3 SEL":i32[](array[numeric])=[0, 2, 3]
  out "Graph S. 4":cluster{dbl[], dbl[]}[](graph)
  out "Graph S. 5":cluster{dbl[], dbl[]}[](graph)
  out "date/time string":string="20190702_164122_"
  out "DAQ OUT \nsample #":u32=1
  in  "DAQ OUT SET Volt":dbl[](array[numeric])=[2.0] format="%0.2f"
  out "Cycle #":i32=68
  out "current time":timestamp=timestamp(3644898422.6679497 s since 1904-01-01)
  in  "?":bool
  in  "Wait (s)":i32=5
  # "Some time needed until program stops!"
  # "Record Config"
  # "VISA address"
  # "Error states"
  # "CH4 of LSI-D broken!"
  # "NI-DAQ config"
  # "Defines # of measurements \n taken for averaging"
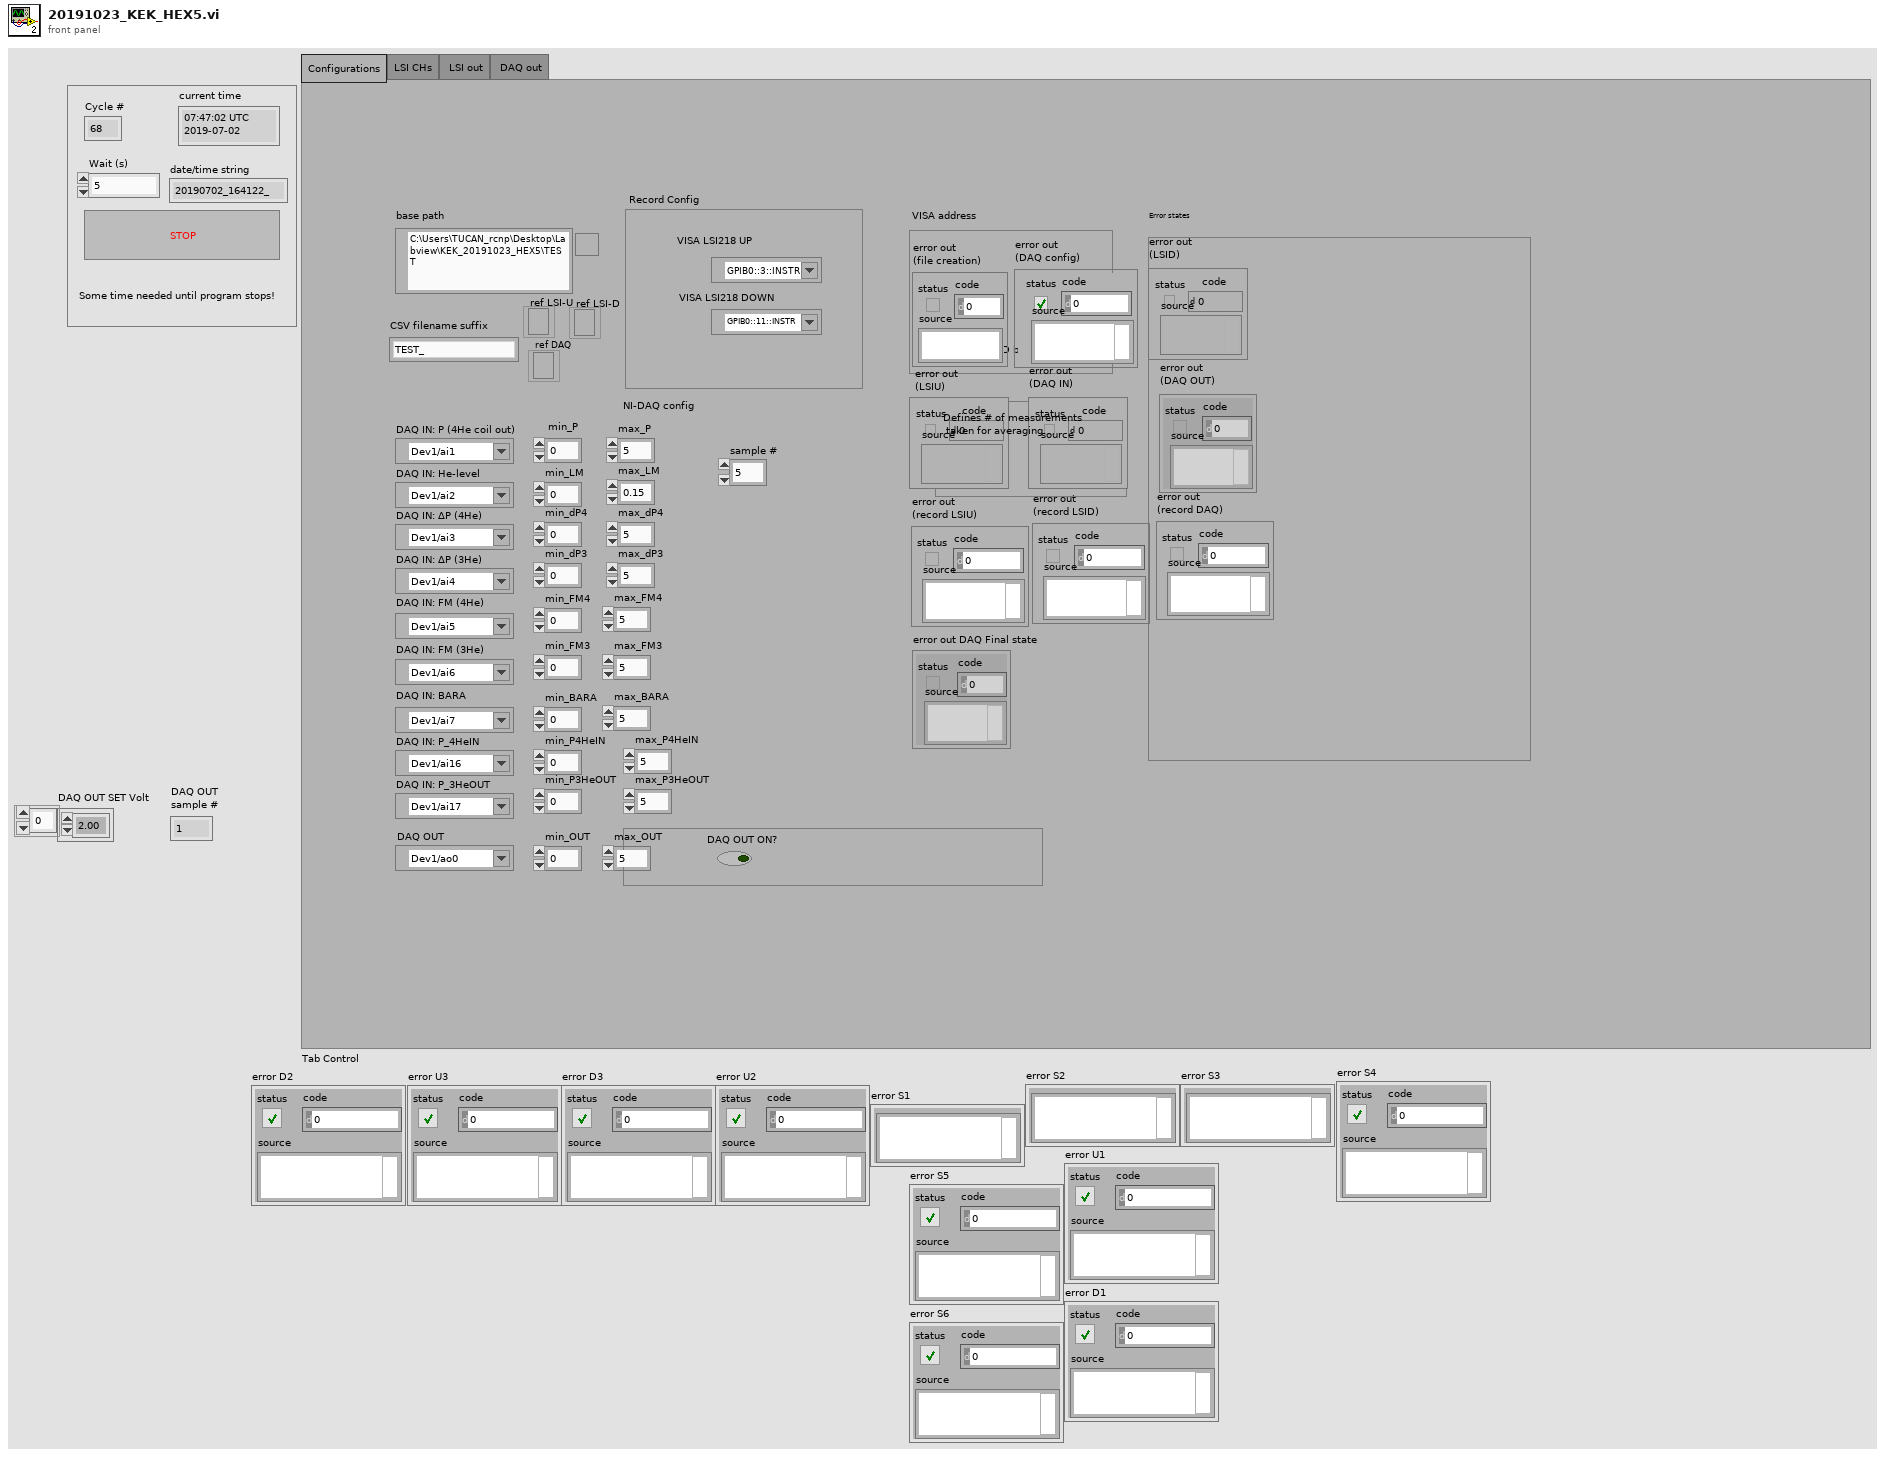
[diagram p1: front panel]
types:
  T1 = enum32{"Configurations", "LSI CHs", " LSI out", " DAQ out"}
  T2 = enum16{"open", "replace", "create", "open or create", "replace or create", "replace or create with confirmation"}
  T3 = cluster{"LSI-U CH labels[0]":string, "LSI-U CH labels[1]":string, "LSI-U CH labels[2]":string, "LSI-U CH labels[3]":string, "LSI-U CH labels[4]":string, "LSI-U CH labels[5]":string, "LSI-U CH labels[6]":string, "LSI-U CH labels[7]":string, "LSI-U CH labels[8]":string}
  T4 = cluster{"LSI-D CH labels[0]":string, "LSI-D CH labels[1]":string, "LSI-D CH labels[2]":string, "LSI-D CH labels[3]":string, "LSI-D CH labels[4]":string, "LSI-D CH labels[5]":string, "LSI-D CH labels[6]":string, "LSI-D CH labels[7]":string, "LSI-D CH labels[8]":string}
  T5 = cluster{"NI DAQ AIN labels[0]":string, "NI DAQ AIN labels[1]":string, "NI DAQ AIN labels[2]":string, "NI DAQ AIN labels[3]":string, "NI DAQ AIN labels[4]":string, "NI DAQ AIN labels[5]":string, "NI DAQ AIN labels[6]":string, "NI DAQ AIN labels[7]":string, "NI DAQ AIN labels[8]":string}
  T6 = cluster{"LSI-D out[0]":dbl, "LSI-D out[1]":dbl, "LSI-D out[2]":dbl, "LSI-D out[3]":dbl, "LSI-D out[4]":dbl, "LSI-D out[5]":dbl, "LSI-D out[6]":dbl, "LSI-D out[7]":dbl, "LSI-D out[8]":dbl}
  T7 = cluster{"LSI-U out[0]":dbl, "LSI-U out[1]":dbl, "LSI-U out[2]":dbl, "LSI-U out[3]":dbl, "LSI-U out[4]":dbl, "LSI-U out[5]":dbl, "LSI-U out[6]":dbl, "LSI-U out[7]":dbl, "LSI-U out[8]":dbl}
  T8 = cluster{"[0]":dbl, "[1]":dbl, "[2]":dbl, "[3]":dbl, "[4]":dbl, "[5]":dbl, "[6]":dbl, "[7]":dbl, "[8]":dbl}
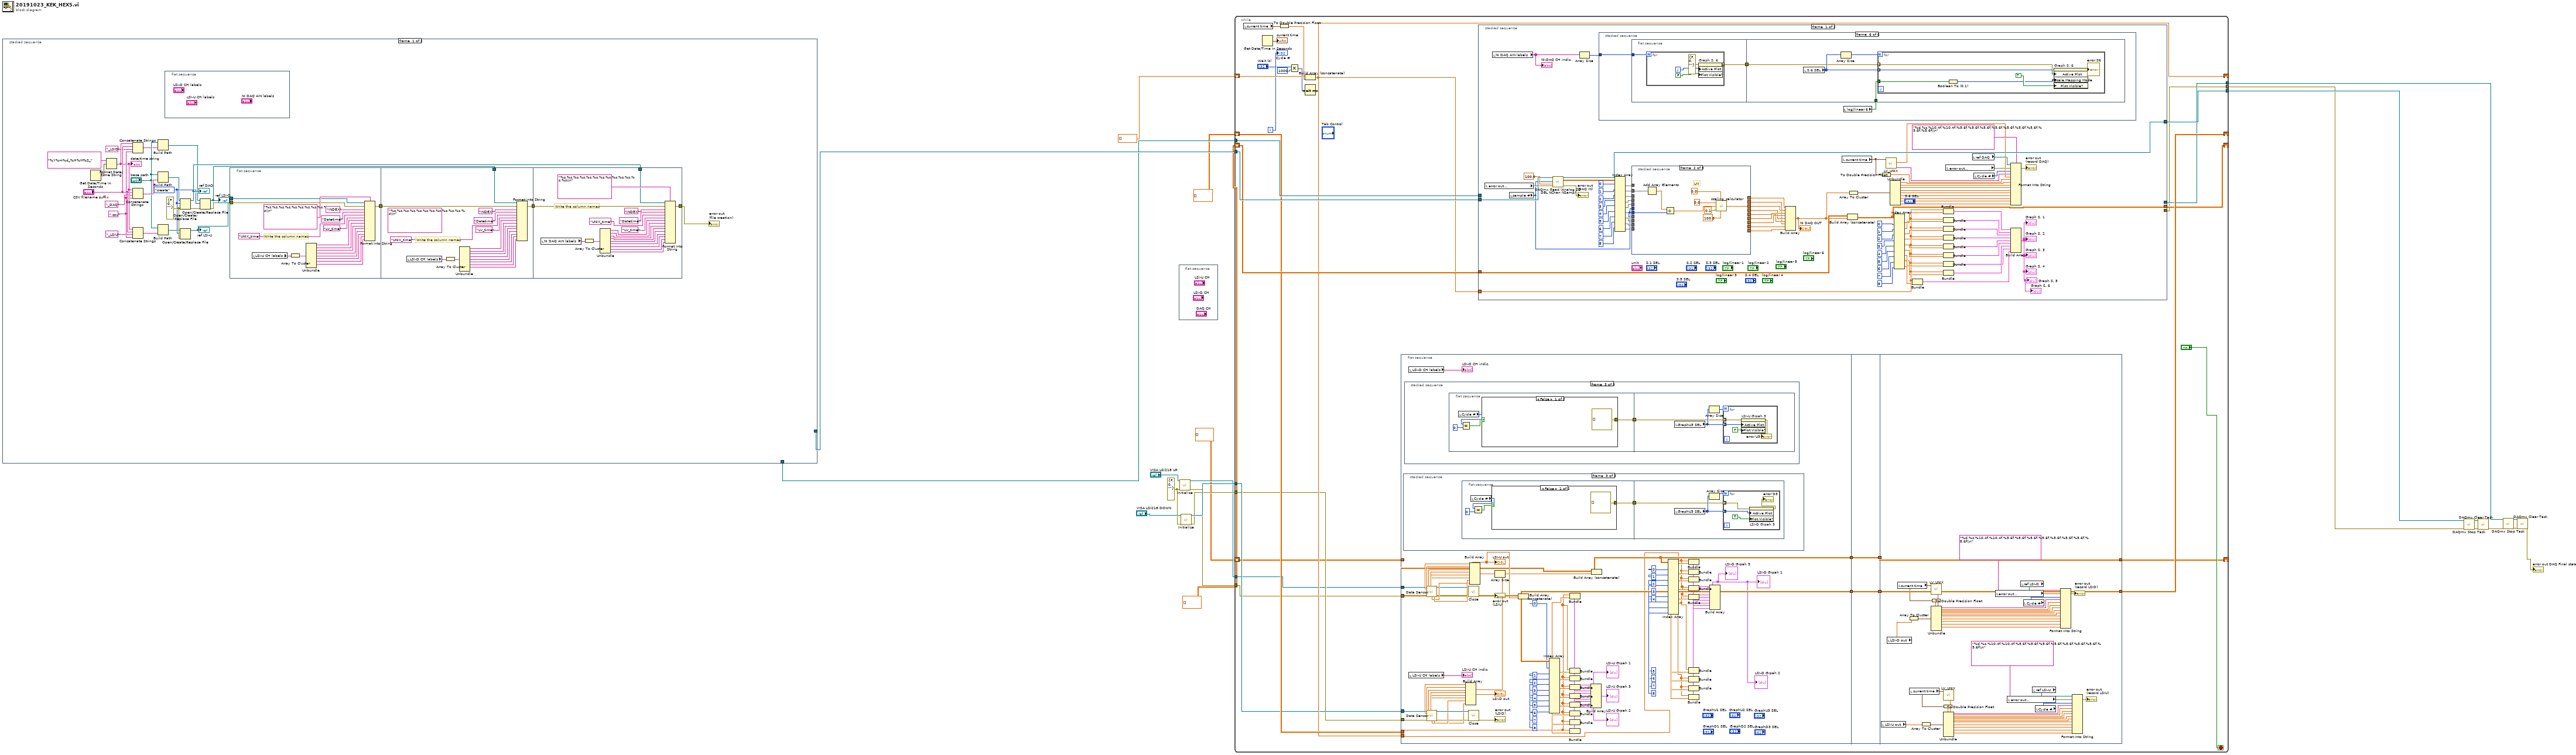
[diagram p0: block diagram]
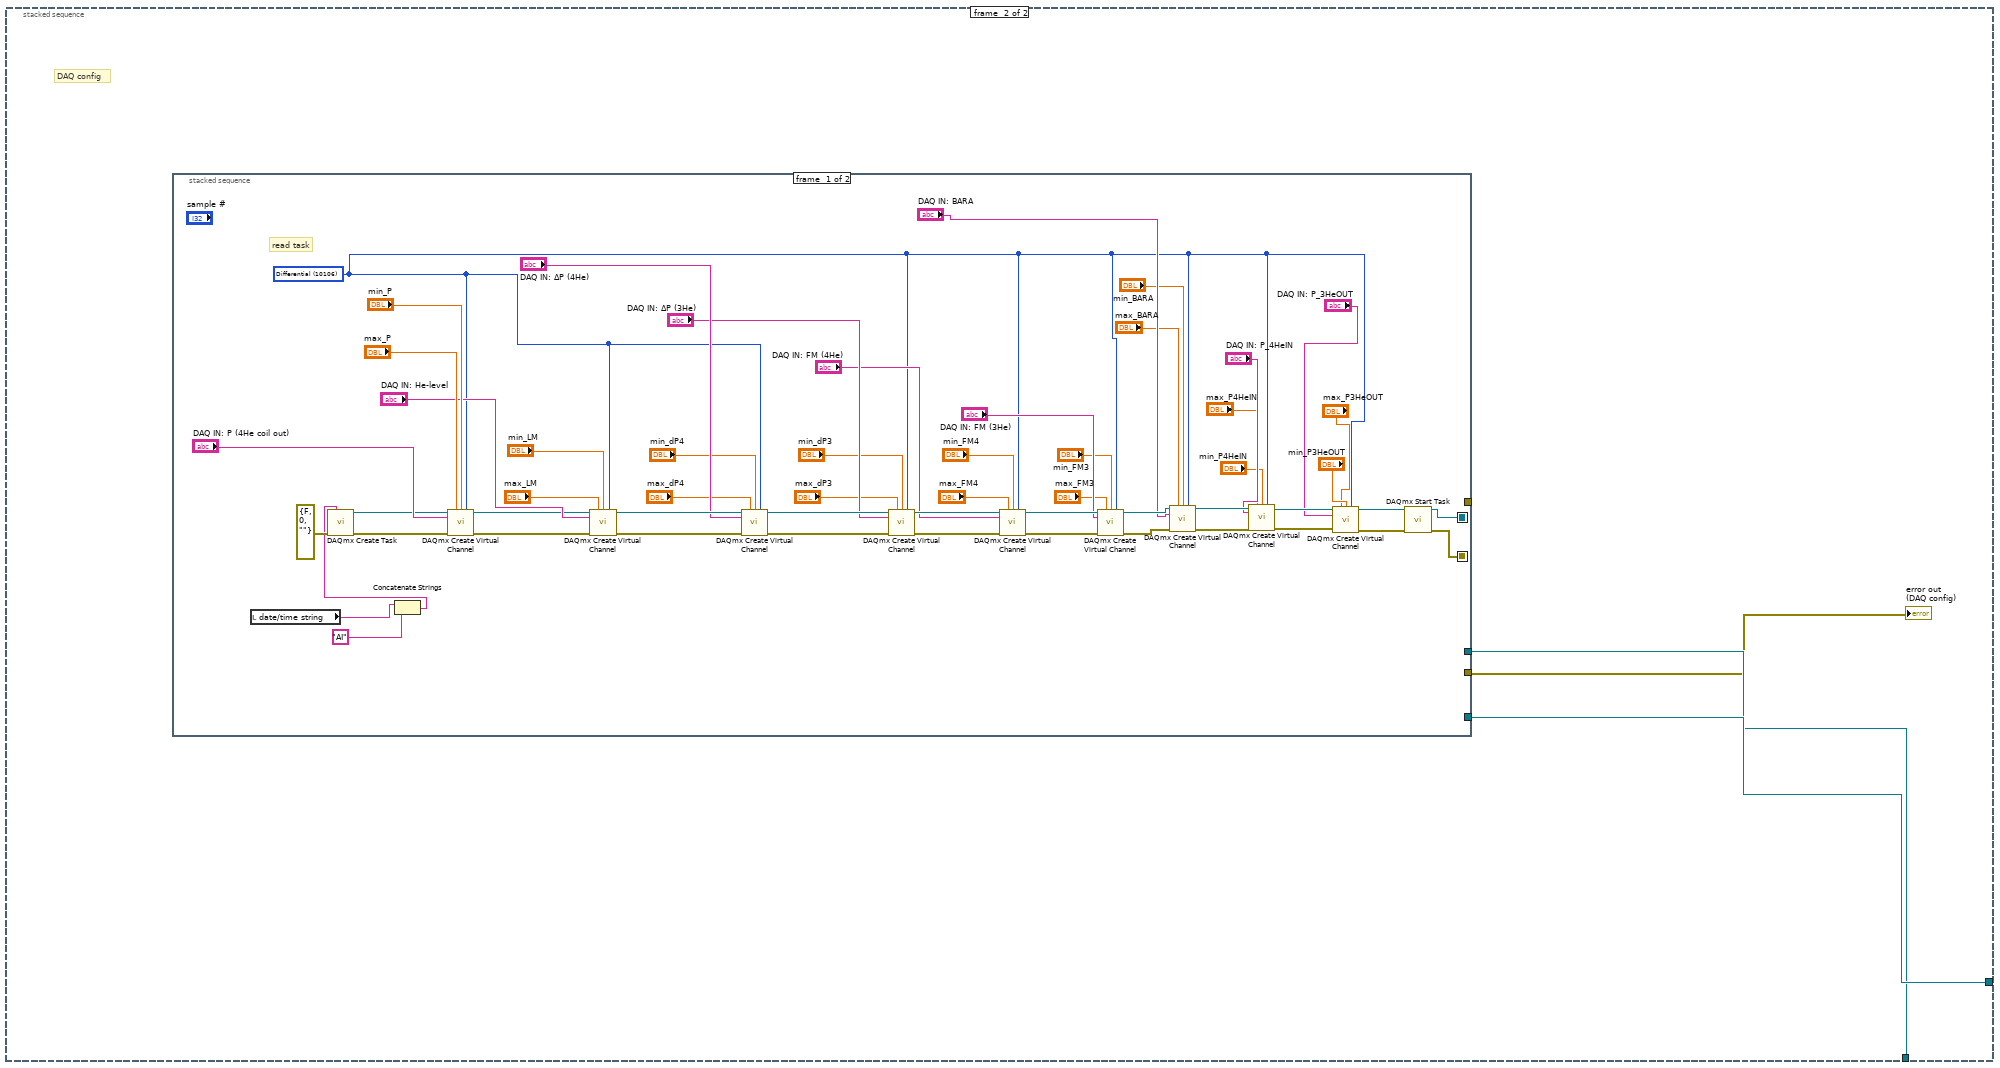
[diagram p2: hidden frame]
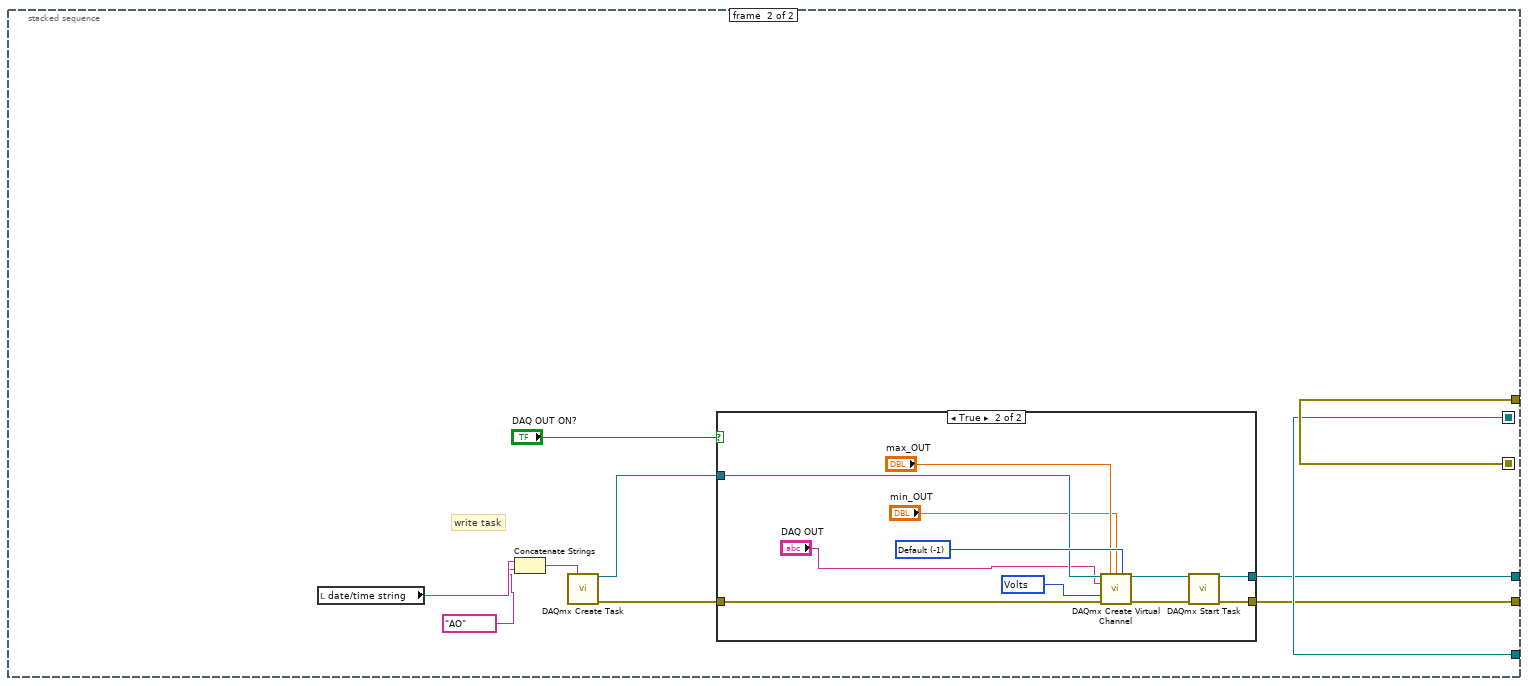
[diagram p3: hidden frame]
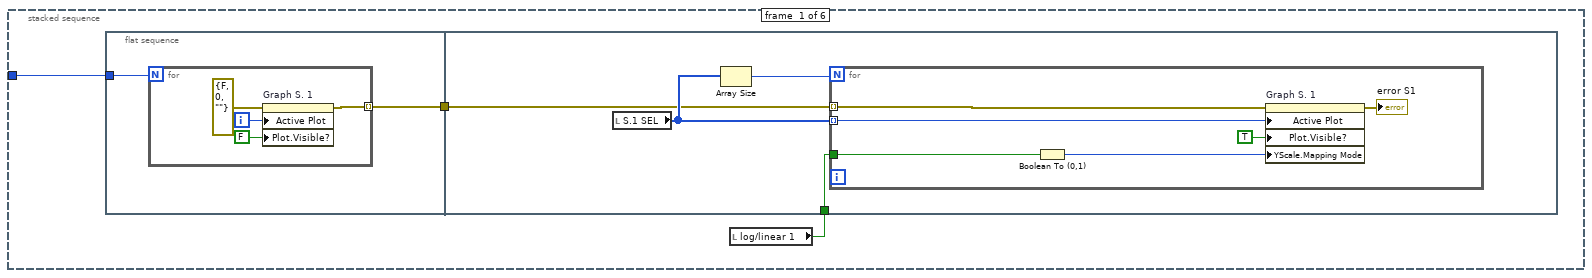
[diagram p5: hidden frame]
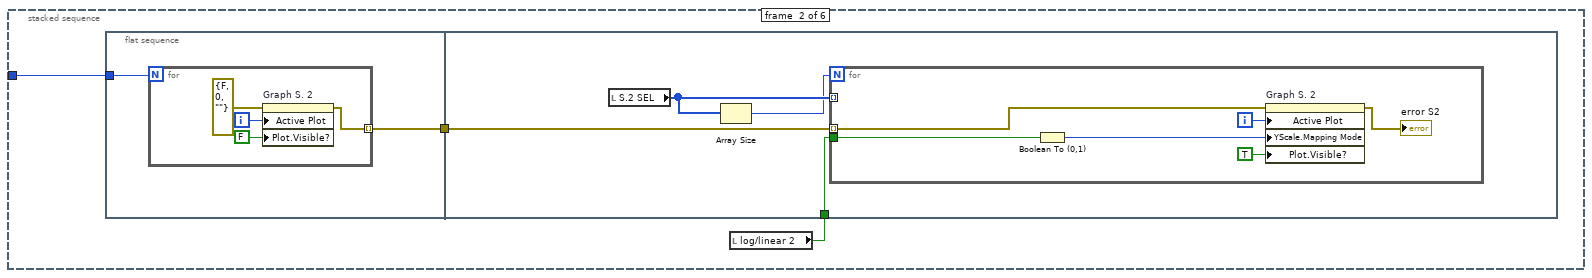
[diagram p6: hidden frame]
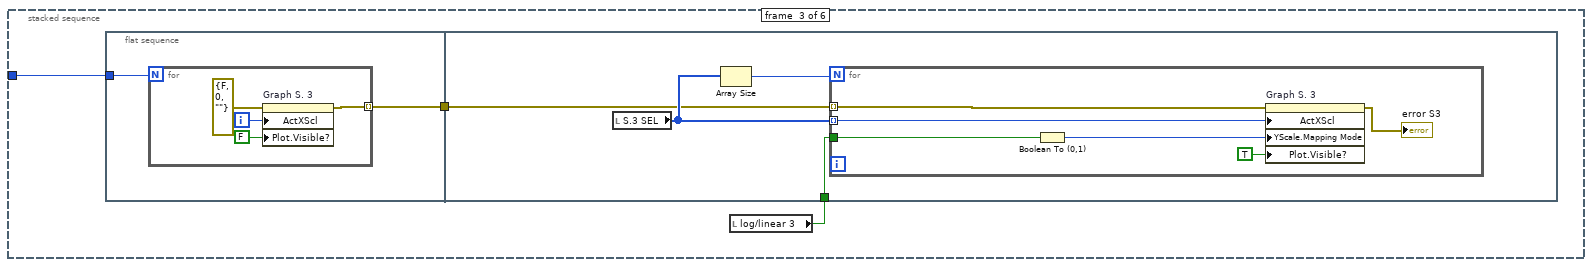
[diagram p7: hidden frame]
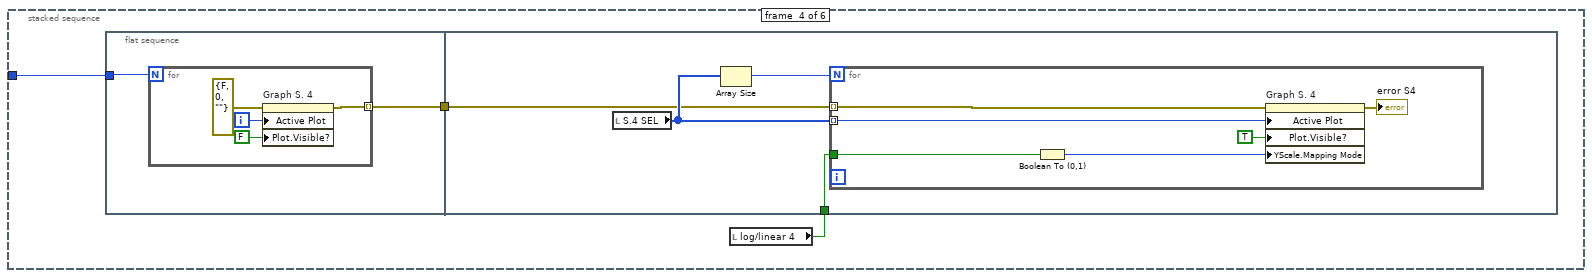
[diagram p8: hidden frame]
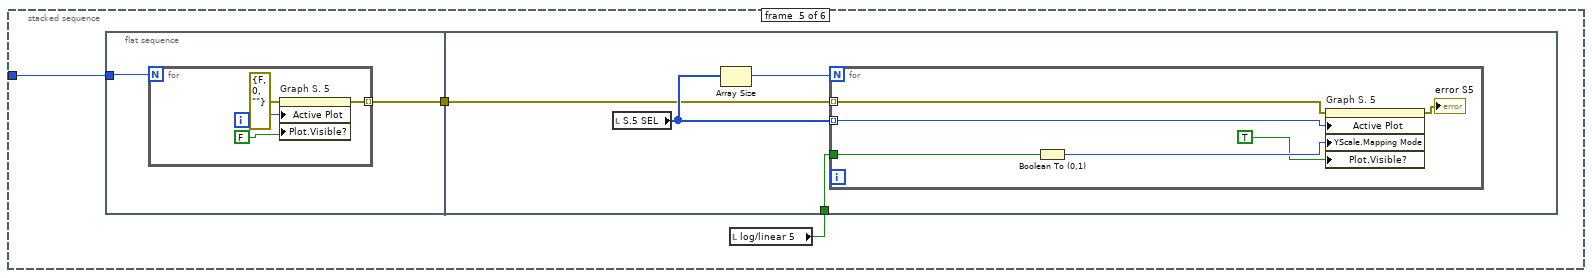
[diagram p9: hidden frame]
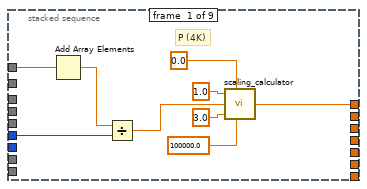
[diagram p10: hidden frame]
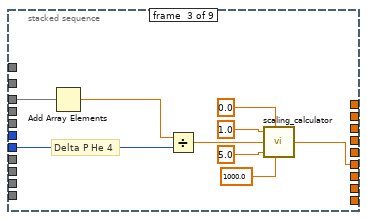
[diagram p11: hidden frame]
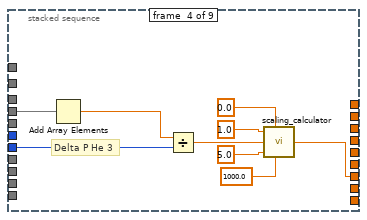
[diagram p12: hidden frame]
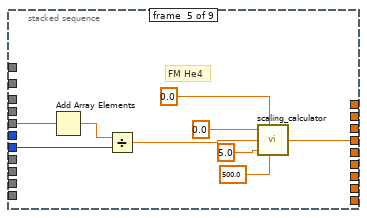
[diagram p13: hidden frame]
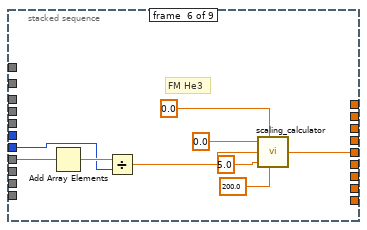
[diagram p14: hidden frame]
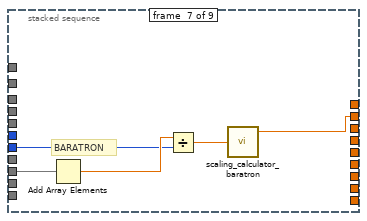
[diagram p15: hidden frame]
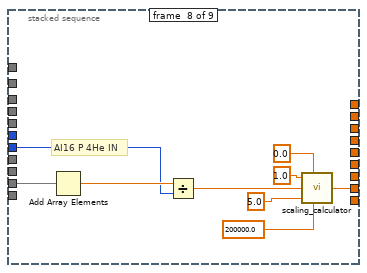
[diagram p16: hidden frame]
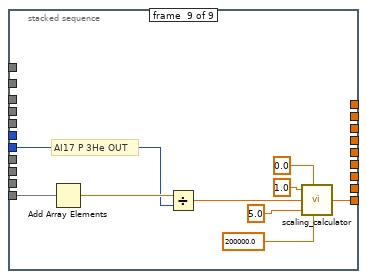
[diagram p17: hidden frame]
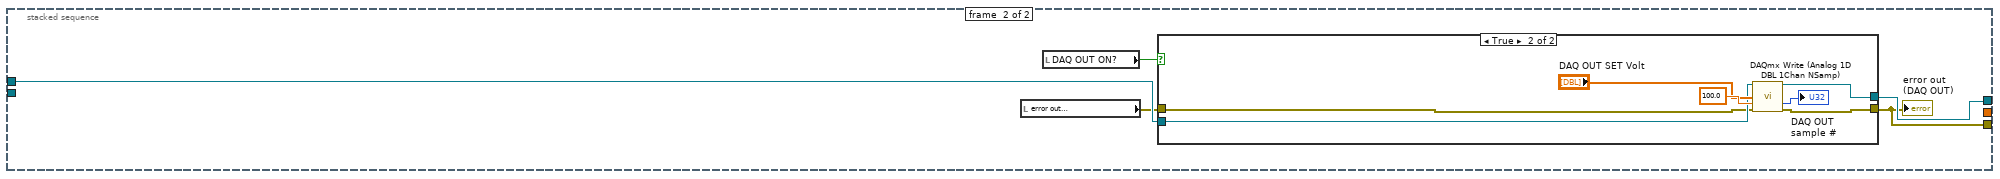
[diagram p18: hidden frame]
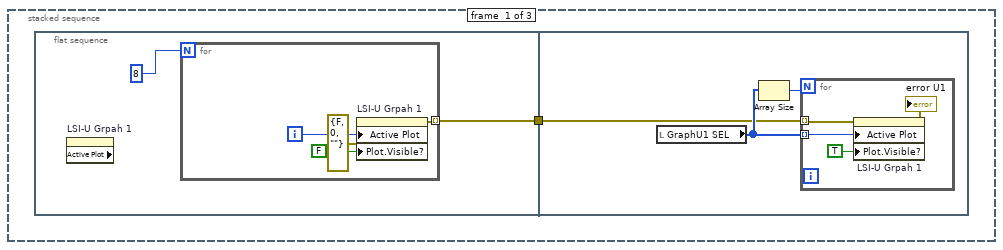
[diagram p20: hidden frame]
diagram:
  w6 = errorcluster {"status"=FALSE, "code"=0, "source"=""} ("error in (no error)")
  n1 = stacked-sequence {
    tunnel: [_ w104] -> w22
    tunnel: [_ w103] -> w21
    frame #0 {
      w39 = errorcluster {"status"=FALSE, "code"=0, "source"=""} ("error in")
      w32 = ".csv" ("string")
      w31 = T2."create" ("operation (0:open)")
      n2 = Get Date/Time In Seconds() -> (seconds since 1Jan1904=w47:timestamp)
      n3 = Format Date/Time String(time format string (%c)="%Y%m%d_%H%M%S_", seconds (now)=w47) -> (date/time string=w35:string)  [unwired: 1 in]
      "date/time string" <- w35
      n4 = Concatenate Strings(w35, "CSV filename suffix", "_LSID" ("string"), w32) -> (w29:string)
      n5 = Concatenate Strings(w35, "CSV filename suffix", "_DAQ" ("string"), w32) -> (w42:string)
      n6 = Concatenate Strings(w35, "CSV filename suffix", "_LSIU" ("string"), w32) -> (w44:string)
      n7 = Build Path(base path="base path", name or relative path=w29) -> (appended path=w28:path)
      n8 = Build Path(base path="base path", name or relative path=w42) -> (appended path=w40:path)
      n9 = Build Path(base path="base path", name or relative path=w44) -> (appended path=w45:path)
      n10 = flat-sequence {
        frame #0 {
        }
      }
      n11 = Open/Create/Replace File(file path (use dialog)=w40, error in=w39, operation (0:open)=w31) -> (refnum out=w37:refnum<file>, error out=w27:errorcluster)  [unwired: 3 in, 1 out]
      "ref DAQ" <- w37
      n12 = Open/Create/Replace File(file path (use dialog)=w45, error in=w39, operation (0:open)=w31) -> (refnum out=w38:refnum<file>)  [unwired: 3 in, 2 out]
      "ref LSI-U" <- w38
      n13 = Open/Create/Replace File(file path (use dialog)=w28, error in=w27, operation (0:open)=w31) -> (refnum out=w23:refnum<file>, error out=w26:errorcluster)  [unwired: 3 in, 1 out]
      "ref LSI-D" <- w23
      n14 = flat-sequence {
        tunnel: w38 -> [w64]
        tunnel: w26 -> [w63]
        tunnel: [w59] -> w25
        tunnel: w25 -> [w68]
        tunnel: [w67] -> w24
        tunnel: w23 -> [w66]
        tunnel: w24 -> [w97]
        tunnel: w37 -> [w96]
        tunnel: [w95] -> w36
        frame #0 {
          # "Write the column names"
          n15 = local read "LSI-U CH labels"() -> (w57:string[])
          n16 = Array To Cluster(array=w57) -> (cluster=w56:T3)
          n17 = Unbundle(w56) -> ("LSI-U CH labels[0]"=w55:string, "LSI-U CH labels[1]"=w54:string, "LSI-U CH labels[2]"=w53:string, "LSI-U CH labels[3]"=w52:string, "LSI-U CH labels[4]"=w51:string, "LSI-U CH labels[5]"=w50:string, "LSI-U CH labels[6]"=w49:string, "LSI-U CH labels[7]"=w48:string)  [unwired: 1 out]
          n18 = Format Into String(format string="%s,%s,%s,%s,%s,%s,%s,%s,%s,%s,%s,%s\\n" ("time format string (%c)"), initial string=w64, error in=w63, "INDEX" ("input 1"), "Datetime" ("input 1"), "UNIX_time" ("input 1"), "LV_time" ("input 1"), w55, w54, w53, w52, w51, w50, w49, w48) -> (error out=w59:errorcluster)  [unwired: 1 out]
        }
        frame #1 {
          (unwired) "%s,%s,%s,%s,%s,%s,%s,%s,%s,%s,%s,%s\\n" ("time format string (%c)")
          # "Write the column names"
          n19 = local read "LSI-D CH labels"() -> (w73:string[])
          n20 = Array To Cluster(array=w73) -> (cluster=w74:T4)
          n21 = Unbundle(w74) -> ("LSI-D CH labels[0]"=w75:string, "LSI-D CH labels[1]"=w76:string, "LSI-D CH labels[2]"=w77:string, "LSI-D CH labels[3]"=w78:string, "LSI-D CH labels[4]"=w79:string, "LSI-D CH labels[5]"=w80:string, "LSI-D CH labels[6]"=w81:string, "LSI-D CH labels[7]"=w82:string)  [unwired: 1 out]
          n22 = Format Into String(initial string=w66, error in=w68, "INDEX" ("input 1"), "Datetime" ("input 1"), "UNIX_time" ("input 1"), "LV_time" ("input 1"), w75, w76, w77, w78, w79, w80, w81, w82) -> (error out=w67:errorcluster)  [unwired: 1 in, 1 out]
        }
        frame #2 {
          # "Write the column names"
          n23 = local read "NI DAQ AIN labels"() -> (w93:string[])
          n24 = Array To Cluster(array=w93) -> (cluster=w92:T5)
          n25 = Unbundle(w92) -> ("NI DAQ AIN labels[0]"=w91:string, "NI DAQ AIN labels[1]"=w90:string, "NI DAQ AIN labels[2]"=w89:string, "NI DAQ AIN labels[3]"=w88:string, "NI DAQ AIN labels[4]"=w87:string, "NI DAQ AIN labels[5]"=w86:string, "NI DAQ AIN labels[6]"=w85:string, "NI DAQ AIN labels[7]"=w84:string, "NI DAQ AIN labels[8]"=w83:string)
          n26 = Format Into String(format string="%s,%s,%s,%s,%s,%s,%s,%s,%s,%s,%s,%s,%s\\n" ("time format string (%c)"), initial string=w96, error in=w97, "INDEX" ("input 1"), "Datetime" ("input 1"), "UNIX_time" ("input 1"), "LV_time" ("input 1"), w91, w90, w89, w88, w87, w86, w85, w84, w83) -> (error out=w95:errorcluster)  [unwired: 1 out]
        }
      }
      "error out\n(file creation)" <- w36
    }
    frame #1 {
      # "DAQ config"
      n27 = stacked-sequence {
        seq-local: [w153 _] -> [_ w168]
        seq-local: [w152 _] -> [_ w167]
        tunnel: [_ w168] -> _
        tunnel: [_ w167] -> w104
        tunnel: [_ w166] -> w103
        tunnel: [_ w165] -> w102
        frame #0 {
          w105 = 10106 items=["Default"=-1, "RSE"=10083, "NRSE"=10078, "Differential"=10106, "Pseudodifferential"=12529] ("input terminal configuration")
          # "read task"
          n28 = local read "date/time string"() -> (w125:string)
          n29 = Concatenate Strings(w125, "AI" ("new task name")) -> (w123:string)
          n30 = call <vilib>:"DAQmx Create Task.vi"("new task name"=w123, "error in"=errorcluster {"status"=FALSE, "code"=0, "source"=""}) -> ("task out"=w154:refnum<k21>, "error out"=w156:errorcluster)  [unwired: 12 in]
          n31 = call-poly <vilib>:"DAQmx Create Virtual Channel.vi"("task in"=w154, "maximum value"="max_P", "minimum value"="min_P", "input terminal configuration"=w105, "physical channels"="DAQ IN: P (4He coil out)", "error in"=w156) -> ("task out"=w146:refnum<k21>, "error out"=w155:errorcluster)  [unwired: 8 in]
          n32 = call-poly <vilib>:"DAQmx Create Virtual Channel.vi"("task in"=w146, "maximum value"="max_LM", "minimum value"="min_LM", "input terminal configuration"=w105, "physical channels"="DAQ IN: He-level", "error in"=w155) -> ("task out"=w143:refnum<k21>, "error out"=w136:errorcluster)  [unwired: 8 in]
          n33 = call-poly <vilib>:"DAQmx Create Virtual Channel.vi"("task in"=w143, "maximum value"="max_dP4", "minimum value"="min_dP4", "input terminal configuration"=w105, "physical channels"="DAQ IN: ΔP (4He)", "error in"=w136) -> ("task out"=w149:refnum<k21>, "error out"=w148:errorcluster)  [unwired: 8 in]
          n34 = call-poly <vilib>:"DAQmx Create Virtual Channel.vi"("task in"=w149, "maximum value"="max_dP3", "minimum value"="min_dP3", "input terminal configuration"=w105, "physical channels"="DAQ IN: ΔP (3He)", "error in"=w148) -> ("task out"=w138:refnum<k21>, "error out"=w135:errorcluster)  [unwired: 8 in]
          n35 = call-poly <vilib>:"DAQmx Create Virtual Channel.vi"("task in"=w138, "maximum value"="max_FM4", "minimum value"="min_FM4", "input terminal configuration"=w105, "physical channels"="DAQ IN: FM (4He)", "error in"=w135) -> ("task out"=w130:refnum<k21>, "error out"=w128:errorcluster)  [unwired: 8 in]
          n36 = call-poly <vilib>:"DAQmx Create Virtual Channel.vi"("task in"=w130, "maximum value"="max_FM3", "minimum value"="min_FM3", "input terminal configuration"=w105, "physical channels"="DAQ IN: FM (3He)", "error in"=w128) -> ("task out"=w121:refnum<k21>, "error out"=w122:errorcluster)  [unwired: 8 in]
          n37 = call-poly <vilib>:"DAQmx Create Virtual Channel.vi"("task in"=w121, "maximum value"="max_BARA", "minimum value"="min_BARA", "input terminal configuration"=w105, "physical channels"="DAQ IN: BARA", "error in"=w122) -> ("task out"=w117:refnum<k21>, "error out"=w116:errorcluster)  [unwired: 8 in]
          n38 = call-poly <vilib>:"DAQmx Create Virtual Channel.vi"("task in"=w117, "maximum value"="max_P4HeIN", "minimum value"="min_P4HeIN", "input terminal configuration"=w105, "physical channels"="DAQ IN: P_4HeIN", "error in"=w116) -> ("task out"=w108:refnum<k21>, "error out"=w110:errorcluster)  [unwired: 8 in]
          n39 = call-poly <vilib>:"DAQmx Create Virtual Channel.vi"("task in"=w108, "maximum value"="max_P3HeOUT", "minimum value"="min_P3HeOUT", "input terminal configuration"=w105, "physical channels"="DAQ IN: P_3HeOUT", "error in"=w110) -> ("task out"=w112:refnum<k21>, "error out"=w111:errorcluster)  [unwired: 8 in]
          n40 = call <vilib>:"DAQmx Start Task.vi"("task/channels in"=w112, "error in"=w111) -> ("task out"=w152:refnum<k21>, "error out"=w153:errorcluster)  [unwired: 12 in]
        }
        frame #1 {
          # "write task"
          n41 = local read "date/time string"() -> (w161:string)
          n42 = Concatenate Strings(w161, "AO" ("new task name")) -> (w159:string)
          n43 = call <vilib>:"DAQmx Create Task.vi"("new task name"=w159) -> ("task out"=w163:refnum<k21>, "error out"=w162:errorcluster)  [unwired: 13 in]
          n44 = case shown="TRUE" "DAQ OUT ON?" {
            tunnel: [w170 w177] -> w166
            tunnel: [w169 w176] -> w165
            tunnel: w163 -> [w170 w175]
            tunnel: w162 -> [w169 w174]
            frame False {
            }
            frame True {
              w179 = -1 items=["Default"=-1, "RSE"=10083, "Differential"=10106, "Pseudodifferential"=12529] ("output terminal configuration")
              w178 = 10348 items=["Volts"=10348, "From Custom Scale"=10065] ("units")
              n45 = call-poly <vilib>:"DAQmx Create Virtual Channel.vi"("task in"=w175, "maximum value"="max_OUT", "minimum value"="min_OUT", "output terminal configuration"=w179, "physical channels"="DAQ OUT", "units"=w178, "error in"=w174) -> ("task out"=w181:refnum<k21>, "error out"=w180:errorcluster)  [unwired: 7 in]
              n46 = call <vilib>:"DAQmx Start Task.vi"("task/channels in"=w181, "error in"=w180) -> ("task out"=w177:refnum<k21>, "error out"=w176:errorcluster)  [unwired: 12 in]
            }
          }
        }
      }
      "error out\n(DAQ config)" <- w102
    }
  }
  n47 = flat-sequence {
    frame #0 {
    }
  }
  n48 = call "Initialize.vi"("VISA resource name"="VISA LSI218 UP", "error in (no error)"=w6) -> ("VISA resource name out"=w3:refnum<visa-resource-name>, "error out"=w2:errorcluster)  [unwired: 12 in]
  n49 = call "Initialize.vi"("VISA resource name"="VISA LSI218 DOWN", "error in (no error)"=w6) -> ("VISA resource name out"=w5:refnum<visa-resource-name>, "error out"=w4:errorcluster)  [unwired: 12 in]
  n50 = while {
    shift-right: [w197] -> _
    shift-left: dbl[] [] -> [w208]
    shift-right: [w200] -> _
    shift-left: dbl[][] [] -> [w201]
    tunnel: w22 -> [w204]
    tunnel: w21 -> [w203]
    shift-right: [w196] -> _
    shift-left: dbl[][] [] -> [w202]
    tunnel: [w192] -> w11
    tunnel: [w191] -> w10
    tunnel: [w190] -> w9
    tunnel: w5 -> [w189]
    tunnel: w4 -> [w188]
    tunnel: w3 -> [w187]
    tunnel: w2 -> [w186]
    shift-right: [w183] -> _
    shift-left: dbl[][] [] -> [w182]
    i -> [w205]
    stop <- "?" stop-if-true
    n51 = local read "current time"() -> (w206:timestamp)
    n52 = Get Date/Time In Seconds() -> (seconds since 1Jan1904=→"current time":timestamp)
    n53 = To Double Precision Float(number=w206) -> (double precision float=w207:dbl)
    n54 = Multiply(x="Wait (s)", y=1000) -> (x*y=w193:i32)
    n55 = Build Array (concatenate)(w208, w207) -> (w197:dbl[])
    n56 = Wait (ms)(milliseconds to wait=w193) -> ()  [unwired: 1 out]
    n57 = flat-sequence {
      tunnel: w197 -> [w504]
      tunnel: w201 -> [w583]
      tunnel: [w572] -> w198
      tunnel: w189 -> [w579]
      tunnel: w188 -> [w578]
      tunnel: w187 -> [w577]
      tunnel: w186 -> [w576]
      tunnel: [w505] -> w184
      tunnel: w182 -> [w506]
      tunnel: [w689] -> w199
      tunnel: w198 -> [w689]
      tunnel: [w688] -> w185
      tunnel: w184 -> [w688]
      tunnel: [w714] -> w200
      tunnel: w199 -> [w714]
      tunnel: [w709] -> w183
      tunnel: w185 -> [w709]
      frame #0 {
        n58 = stacked-sequence {
          frame #0 {
            n59 = flat-sequence {
              tunnel: [w642] -> w641
              tunnel: w641 -> [w648]
              frame #0 {
                n60 = for {
                  N: 8 -> [_]
                  tunnel: [w644] -> w642 mode=indexing
                  i -> [w647]
                  n61 = property on="LSI-D Grpah 1" class="XYGraph （指定）"(error in=errorcluster {"status"=FALSE, "code"=0, "source"=""} ("error in (no error)"), "Active Plot"=w647, "Plot.Visible?"=FALSE ("Plot.Visible")) -> (error out=w644:errorcluster)  [unwired: 1 in, 1 out]
                }
              }
              frame #1 {
                n62 = local read "GraphU1 SEL"() -> (w649:i32[])
                n63 = Array Size(array=w649) -> (size(s)=w650:i32)
                n64 = for {
                  N: w650 -> [_]
                  tunnel: w649 -> [w654] mode=indexing
                  tunnel: w648 -> [w652] mode=indexing
                  n65 = property on="LSI-D Grpah 1" class="XYGraph （指定）"(error in=w652, "Active Plot"=w654, "Plot.Visible?"=TRUE ("Plot.Visible")) -> (error out=→"error D1":errorcluster)  [unwired: 1 in, 1 out]
                }
              }
            }
          }
          frame #1 {
            n66 = flat-sequence {
              tunnel: [w656] -> w655
              tunnel: w655 -> [w662]
              frame #0 {
                n67 = for {
                  N: 8 -> [_]
                  tunnel: [w659] -> w656 mode=indexing
                  i -> [w661]
                  n68 = property on="LSI-D Grpah 2" class="XYGraph （指定）"(error in=errorcluster {"status"=FALSE, "code"=0, "source"=""} ("error in (no error)"), "Active Plot"=w661, "Plot.Visible?"=FALSE ("Plot.Visible")) -> (error out=w659:errorcluster)  [unwired: 1 in, 1 out]
                }
              }
              frame #1 {
                n69 = local read "GraphU2 SEL"() -> (w663:i32[])
                n70 = Array Size(array=w663) -> (size(s)=w664:i32)
                n71 = for {
                  N: w664 -> [_]
                  tunnel: w663 -> [w668] mode=indexing
                  tunnel: w662 -> [w665] mode=indexing
                  n72 = property on="LSI-D Grpah 2" class="XYGraph （指定）"(error in=w665, "Active Plot"=w668, "Plot.Visible?"=TRUE ("Plot.Visible")) -> (error out=→"error D2":errorcluster)  [unwired: 1 in, 1 out]
                }
              }
            }
          }
          frame #2 {
            n73 = flat-sequence {
              tunnel: [w673] -> w669
              tunnel: w669 -> [w681]
              frame #0 {
                n74 = local read "Cycle #"() -> (w671:i32)
                n75 = Equal?(x=w671, y=0) -> (x = y?=w670:bool)
                n76 = case shown="FALSE" w670 {
                  tunnel: [errorcluster[] [] w675] -> w673
                  frame False {
                  }
                  frame True {
                    n77 = for {
                      N: 8 -> [_]
                      tunnel: [w677] -> w675 mode=indexing
                      i -> [w680]
                      n78 = property on="LSI-D Grpah 3" class="XYGraph （指定）"(error in=errorcluster {"status"=FALSE, "code"=0, "source"=""} ("error in (no error)"), "Active Plot"=w680, "Plot.Visible?"=FALSE ("Plot.Visible")) -> (error out=w677:errorcluster)  [unwired: 1 in, 1 out]
                    }
                  }
                }
              }
              frame #1 {
                n79 = local read "GraphU3 SEL"() -> (w682:i32[])
                n80 = Array Size(array=w682) -> (size(s)=w683:i32)
                n81 = for {
                  N: w683 -> [_]
                  tunnel: w682 -> [w687] mode=indexing
                  tunnel: w681 -> [w685] mode=indexing
                  n82 = property on="LSI-D Grpah 3" class="XYGraph （指定）"(error in=w685, "Active Plot"=w687, "Plot.Visible?"=TRUE ("Plot.Visible")) -> (error out=→"error D3":errorcluster)  [unwired: 1 in, 1 out]
                }
              }
            }
          }
        }
        n83 = stacked-sequence {
          frame #0 {
            n84 = flat-sequence {
              tunnel: [w595] -> w594
              tunnel: w594 -> [w601]
              frame #0 {
                n85 = property on="LSI-U Grpah 1" class="XYGraph （指定）" props=["Active Plot"]() -> ()  [unwired: 2 in, 3 out]
                n86 = for {
                  N: 8 -> [_]
                  tunnel: [w597] -> w595 mode=indexing
                  i -> [w599]
                  n87 = property on="LSI-U Grpah 1" class="XYGraph （指定）"(error in=errorcluster {"status"=FALSE, "code"=0, "source"=""} ("error in (no error)"), "Active Plot"=w599, "Plot.Visible?"=FALSE ("Plot.Visible")) -> (error out=w597:errorcluster)  [unwired: 1 in, 1 out]
                }
              }
              frame #1 {
                n88 = local read "GraphU1 SEL"() -> (w602:i32[])
                n89 = Array Size(array=w602) -> (size(s)=w603:i32)
                n90 = for {
                  N: w603 -> [_]
                  tunnel: w602 -> [w606] mode=indexing
                  tunnel: w601 -> [w605] mode=indexing
                  n91 = property on="LSI-U Grpah 1" class="XYGraph （指定）"(error in=w605, "Active Plot"=w606, "Plot.Visible?"=TRUE ("Plot.Visible")) -> (error out=→"error U1":errorcluster)  [unwired: 1 in, 1 out]
                }
              }
            }
          }
          frame #1 {
            n92 = flat-sequence {
              tunnel: [w609] -> w608
              tunnel: w608 -> [w615]
              frame #0 {
                n93 = for {
                  N: 8 -> [_]
                  tunnel: [w611] -> w609 mode=indexing
                  i -> [w614]
                  n94 = property on="LSI-U Grpah 2" class="XYGraph （指定）"(error in=errorcluster {"status"=FALSE, "code"=0, "source"=""} ("error in (no error)"), "Active Plot"=w614, "Plot.Visible?"=FALSE ("Plot.Visible")) -> (error out=w611:errorcluster)  [unwired: 1 in, 1 out]
                }
              }
              frame #1 {
                n95 = local read "GraphU2 SEL"() -> (w616:i32[])
                n96 = Array Size(array=w616) -> (size(s)=w617:i32)
                n97 = for {
                  N: w617 -> [_]
                  tunnel: w616 -> [w620] mode=indexing
                  tunnel: w615 -> [w619] mode=indexing
                  n98 = property on="LSI-U Grpah 2" class="XYGraph （指定）"(error in=w619, "Active Plot"=w620, "Plot.Visible?"=TRUE ("Plot.Visible")) -> (error out=→"error U2":errorcluster)  [unwired: 1 in, 1 out]
                }
              }
            }
          }
          frame #2 {
            n99 = flat-sequence {
              tunnel: [w626] -> w622
              tunnel: w622 -> [w634]
              frame #0 {
                n100 = local read "Cycle #"() -> (w625:i32)
                n101 = Equal?(x=w625, y=0) -> (x = y?=w623:bool)
                n102 = case shown="FALSE" w623 {
                  tunnel: [errorcluster[] [] w628] -> w626
                  frame False {
                  }
                  frame True {
                    n103 = for {
                      N: 8 -> [_]
                      tunnel: [w630] -> w628 mode=indexing
                      i -> [w632]
                      n104 = property on="LSI-U Grpah 3" class="XYGraph （指定）"(error in=errorcluster {"status"=FALSE, "code"=0, "source"=""} ("error in (no error)"), "Active Plot"=w632, "Plot.Visible?"=FALSE ("Plot.Visible")) -> (error out=w630:errorcluster)  [unwired: 1 in, 1 out]
                    }
                  }
                }
              }
              frame #1 {
                n105 = local read "GraphU3 SEL"() -> (w635:i32[])
                n106 = Array Size(array=w635) -> (size(s)=w636:i32)
                n107 = for {
                  N: w636 -> [_]
                  tunnel: w635 -> [w640] mode=indexing
                  tunnel: w634 -> [w638] mode=indexing
                  n108 = property on="LSI-U Grpah 3" class="XYGraph （指定）"(error in=w638, "Active Plot"=w640, "Plot.Visible?"=TRUE ("Plot.Visible")) -> (error out=→"error U3":errorcluster)  [unwired: 1 in, 1 out]
                }
              }
            }
          }
        }
        n109 = local read "LSI-D CH labels"() -> (→"LSI-D CH indic.":string[])
        n110 = local read "LSI-U CH labels"() -> (→"LSI-U CH indic,":string[])
        n111 = call "Data Sensor.vi"("VISA resource name"=w577, "error in (no error)"=w576) -> ("Input 1"=w593:dbl, "Input 2"=w592:dbl, "Input 3"=w591:dbl, "VISA resource name out"=w585:refnum<visa-resource-name>, "Input 4"=w575:dbl, "Input 5"=w590:dbl, "Input 6"=w589:dbl, "Input 8"=w587:dbl, "Input 7"=w588:dbl, "error out"=w586:errorcluster)  [unwired: 4 in]
        n112 = call "Data Sensor.vi"("VISA resource name"=w579, "error in (no error)"=w578) -> ("Input 1"=w543:dbl, "Input 2"=w542:dbl, "Input 3"=w541:dbl, "VISA resource name out"=w581:refnum<visa-resource-name>, "Input 4"=w540:dbl, "Input 5"=w539:dbl, "Input 6"=w538:dbl, "Input 8"=w536:dbl, "Input 7"=w537:dbl, "error out"=w580:errorcluster)  [unwired: 4 in]
        n113 = Build Array(w543, w542, w541, w540, w539, w538, w537, w536) -> (w507:dbl[])
        "LSI-D out" <- w507
        n114 = call "Close.vi"("VISA resource name"=w585, "error in (no error)"=w586) -> ("error out"=→"error out \n(LSIU)":errorcluster)  [unwired: 13 in]
        n115 = call "Close.vi"("VISA resource name"=w581, "error in (no error)"=w580) -> ("error out"=→"error out \n(LSID)":errorcluster)  [unwired: 13 in]
        n116 = Build Array(w593, w592, w591, w575, w590, w589, w588, w587) -> (w573:dbl[])
        "LSI-U out" <- w573
        n117 = Array Size(array=w573) -> ()  [unwired: 1 out]
        n118 = Build Array (concatenate)(w583, w573) -> (w572:dbl[][])
        n119 = Index Array(array=w572, index (col) #1=0 ("disabled index (col)"), index (col) #2=1 ("index (col)"), index (col) #3=2 ("index (col)"), index (col) #4=3 ("index (col)"), index (col) #5=4 ("index (col)"), index (col) #6=5 ("index (col)"), index (col) #7=6 ("index (col)"), index (col) #8=7 ("index (col)"), index (col) #9=8 ("index (col)")) -> (element #1=w570:dbl[], element #2=w561:dbl[], element #3=w560:dbl[], element #4=w559:dbl[], element #5=w558:dbl[], element #6=w557:dbl[], element #7=w556:dbl[], element #8=w555:dbl[], element #9=w554:dbl[])  [unwired: 9 in]
        n120 = Bundle(w504, w570) -> (w553:cluster{dbl[], dbl[]})  [unwired: 1 in]
        n121 = Bundle(w504, w561) -> (w552:cluster{dbl[], dbl[]})  [unwired: 1 in]
        n122 = Bundle(w504, w560) -> (w551:cluster{dbl[], dbl[]})  [unwired: 1 in]
        n123 = Bundle(w504, w559) -> (w550:cluster{dbl[], dbl[]})  [unwired: 1 in]
        n124 = Bundle(w504, w558) -> (w549:cluster{dbl[], dbl[]})  [unwired: 1 in]
        n125 = Bundle(w504, w557) -> (w548:cluster{dbl[], dbl[]})  [unwired: 1 in]
        n126 = Bundle(w504, w556) -> (w547:cluster{dbl[], dbl[]})  [unwired: 1 in]
        n127 = Bundle(w504, w555) -> (w546:cluster{dbl[], dbl[]})  [unwired: 1 in]
        n128 = Bundle(w504, w554) -> (w545:cluster{dbl[], dbl[]})  [unwired: 1 in]
        n129 = Build Array(w553, w552, w551, w550, w549, w548, w547, w546, w545) -> (→"LSI-U Grpah 1" →"LSI-U Grpah 2" →"LSI-U Grpah 3":cluster{dbl[], dbl[]}[])
        n130 = Build Array (concatenate)(w506, w507) -> (w505:dbl[][])
        n131 = Index Array(array=w505, index (col) #1=0 ("disabled index (col)"), index (col) #2=1 ("index (col)"), index (col) #3=2 ("index (col)"), index (col) #4=3 ("index (col)"), index (col) #5=4 ("index (col)"), index (col) #6=5 ("index (col)"), index (col) #7=6 ("index (col)"), index (col) #8=7 ("index (col)"), index (col) #9=8 ("index (col)")) -> (element #1=w509:dbl[], element #2=w518:dbl[], element #3=w519:dbl[], element #4=w520:dbl[], element #5=w521:dbl[], element #6=w522:dbl[], element #7=w523:dbl[], element #8=w524:dbl[], element #9=w525:dbl[])  [unwired: 9 in]
        n132 = Bundle(w504, w509) -> (w526:cluster{dbl[], dbl[]})  [unwired: 1 in]
        n133 = Bundle(w504, w518) -> (w527:cluster{dbl[], dbl[]})  [unwired: 1 in]
        n134 = Bundle(w504, w519) -> (w528:cluster{dbl[], dbl[]})  [unwired: 1 in]
        n135 = Bundle(w504, w520) -> (w529:cluster{dbl[], dbl[]})  [unwired: 1 in]
        n136 = Bundle(w504, w521) -> (w530:cluster{dbl[], dbl[]})  [unwired: 1 in]
        n137 = Bundle(w504, w522) -> (w531:cluster{dbl[], dbl[]})  [unwired: 1 in]
        n138 = Bundle(w504, w523) -> (w532:cluster{dbl[], dbl[]})  [unwired: 1 in]
        n139 = Bundle(w504, w524) -> (w533:cluster{dbl[], dbl[]})  [unwired: 1 in]
        n140 = Bundle(w504, w525) -> (w534:cluster{dbl[], dbl[]})  [unwired: 1 in]
        n141 = Build Array(w526, w527, w528, w529, w530, w531, w532, w533, w534) -> (→"LSI-D Grpah 3" →"LSI-D Grpah 2" →"LSI-D Grpah 1":cluster{dbl[], dbl[]}[])
      }
      frame #1 {
      }
      frame #2 {
        n142 = local read "LSI-U out"() -> (w725:dbl[])
        n143 = local read "LSI-D out"() -> (w690:dbl[])
        n144 = local read "current time"() -> (w705:timestamp)
        n145 = Array To Cluster(array=w690) -> (cluster=w695:T6)
        n146 = local read "current time"() -> (w713:timestamp)
        n147 = Array To Cluster(array=w725) -> (cluster=w724:T7)
        n148 = To Double Precision Float(number=w705) -> (double precision float=w693:dbl)
        n149 = call "LV_UNIX.vi"("current time"=w705) -> ("date/time string"=w707:string, "UNIX time (s)"=w706:dbl)  [unwired: 9 in]
        n150 = Unbundle(w695) -> ("LSI-D out[0]"=w696:dbl, "LSI-D out[1]"=w697:dbl, "LSI-D out[2]"=w698:dbl, "LSI-D out[3]"=w699:dbl, "LSI-D out[4]"=w700:dbl, "LSI-D out[5]"=w701:dbl, "LSI-D out[6]"=w702:dbl, "LSI-D out[7]"=w703:dbl)  [unwired: 1 out]
        n151 = To Double Precision Float(number=w713) -> (double precision float=w727:dbl)
        n152 = call "LV_UNIX.vi"("current time"=w713) -> ("date/time string"=w711:string, "UNIX time (s)"=w712:dbl)  [unwired: 9 in]
        n153 = Unbundle(w724) -> ("LSI-U out[0]"=w723:dbl, "LSI-U out[1]"=w722:dbl, "LSI-U out[2]"=w721:dbl, "LSI-U out[3]"=w720:dbl, "LSI-U out[4]"=w719:dbl, "LSI-U out[5]"=w718:dbl, "LSI-U out[6]"=w717:dbl, "LSI-U out[7]"=w716:dbl)  [unwired: 1 out]
        n154 = local read "error out\n(file creation)"() -> (w692:errorcluster)
        n155 = local read "error out\n(file creation)"() -> (w728:errorcluster)
        n156 = local read "ref LSI-D"() -> (w691:refnum<file>)
        n157 = local read "Cycle #"() -> (w708:i32)
        n158 = local read "ref LSI-U"() -> (w729:refnum<file>)
        n159 = local read "Cycle #"() -> (w710:i32)
        n160 = Format Into String(format string="%d,%s,%10.4f,%10.4f,%5.6f,%5.6f,%5.6f,%5.6f,%5.6f,%5.6f,%5.6f,%5.6f\\n", initial string=w691, error in=w692, w708, w707, w706, w693, w696, w697, w698, w699, w700, w701, w702, w703) -> (error out=→"error out \n(record LSID)":errorcluster)  [unwired: 1 out]
        n161 = Format Into String(format string="%d,%s,%10.4f,%10.4f,%5.6f,%5.6f,%5.6f,%5.6f,%5.6f,%5.6f,%5.6f,%5.6f\\n", initial string=w729, error in=w728, w710, w711, w712, w727, w723, w722, w721, w720, w719, w718, w717, w716) -> (error out=→"error out \n(record LSIU)":errorcluster)  [unwired: 1 out]
      }
    }
    n162 = stacked-sequence {
      tunnel: w204 -> [w297 _]
      tunnel: w203 -> [_ w493]
      tunnel: [_ w491] -> w191
      tunnel: w202 -> [w275 _]
      tunnel: [w233 _] -> w196
      tunnel: w197 -> [w232 _]
      tunnel: [w274 _] -> w192
      tunnel: [_ w489] -> w190
      frame #0 {
        n163 = local read "error out\n(DAQ config)"() -> (w293:errorcluster)
        n164 = local read "NI DAQ AIN labels"() -> (w213:string[])
        "NI-DAQ CH indic." <- w213
        n165 = local read "sample #"() -> (w270:i32)
        n166 = call <vilib>:"DAQmx Read (Analog 2D DBL NChan NSamp).vi"("task/channels in"=w297, "number of samples per channel"=w270, "timeout"=100.0, "error in"=w293) -> ("task out"=w274:refnum<k21>, "data"=w292:dbl[][], "error out"=→"error out \n(DAQ IN)":errorcluster)  [unwired: 9 in]
        n167 = Array Size(array=w213) -> (size(s)=w226:i32)
        n168 = stacked-sequence {
          tunnel: w226 -> [w300 w319 w338 w357 w376 w395]
          frame #0 {
            n169 = flat-sequence {
              tunnel: w300 -> [w302]
              tunnel: [w301] -> w298
              tunnel: w299 -> [w310]
              tunnel: w298 -> [w307]
              frame #0 {
                n170 = for {
                  N: w302 -> [_]
                  tunnel: [w303] -> w301 mode=indexing
                  i -> [w306]
                  n171 = property on="Graph S. 1" class="XYGraph （指定）"(error in=errorcluster {"status"=FALSE, "code"=0, "source"=""} ("error in (no error)"), "Active Plot"=w306, "Plot.Visible?"=FALSE ("Plot.Visible")) -> (error out=w303:errorcluster)  [unwired: 1 in, 1 out]
                }
              }
              frame #1 {
                n172 = local read "S.1 SEL"() -> (w309:i32[])
                n173 = Array Size(array=w309) -> (size(s)=w308:i32)
                n174 = for {
                  N: w308 -> [_]
                  tunnel: w309 -> [w316] mode=indexing
                  tunnel: w310 -> [w314]
                  tunnel: w307 -> [w312] mode=indexing
                  n175 = Boolean To (0,1)(Boolean=w314) -> (0, 1=w313:i16)
                  n176 = property on="Graph S. 1" class="XYGraph （指定）"(error in=w312, "Active Plot"=w316, "Plot.Visible?"=TRUE ("Plot.Visible"), "YScale.Mapping Mode"=w313) -> (error out=→"error S1":errorcluster)  [unwired: 1 in, 1 out]
                }
              }
            }
            n177 = local read "log/linear 1"() -> (w299:bool)
          }
          frame #1 {
            n178 = flat-sequence {
              tunnel: w319 -> [w321]
              tunnel: [w320] -> w317
              tunnel: w318 -> [w329]
              tunnel: w317 -> [w326]
              frame #0 {
                n179 = for {
                  N: w321 -> [_]
                  tunnel: [w322] -> w320 mode=indexing
                  i -> [w325]
                  n180 = property on="Graph S. 2" class="XYGraph （指定）"(error in=errorcluster {"status"=FALSE, "code"=0, "source"=""} ("error in (no error)"), "Active Plot"=w325, "Plot.Visible?"=FALSE ("Plot.Visible")) -> (error out=w322:errorcluster)  [unwired: 1 in, 1 out]
                }
              }
              frame #1 {
                n181 = local read "S.2 SEL"() -> (w328:i32[])
                n182 = Array Size(array=w328) -> (size(s)=w327:i32)
                n183 = for {
                  N: w327 -> [_]
                  tunnel: w328 -> [_] mode=indexing
                  tunnel: w329 -> [w335]
                  tunnel: w326 -> [w330] mode=indexing
                  i -> [w332]
                  n184 = Boolean To (0,1)(Boolean=w335) -> (0, 1=w334:i16)
                  n185 = property on="Graph S. 2" class="XYGraph （指定）"(error in=w330, "Active Plot"=w332, "YScale.Mapping Mode"=w334, "Plot.Visible?"=TRUE ("Plot.Visible")) -> (error out=→"error S2":errorcluster)  [unwired: 1 in, 1 out]
                }
              }
            }
            n186 = local read "log/linear 2"() -> (w318:bool)
          }
          frame #2 {
            n187 = flat-sequence {
              tunnel: w338 -> [w340]
              tunnel: [w339] -> w336
              tunnel: w337 -> [w348]
              tunnel: w336 -> [w345]
              frame #0 {
                n188 = for {
                  N: w340 -> [_]
                  tunnel: [w341] -> w339 mode=indexing
                  i -> [w344]
                  n189 = property on="Graph S. 3" class="XYGraph （指定）"(error in=errorcluster {"status"=FALSE, "code"=0, "source"=""} ("error in (no error)"), "ActXScl"=w344, "Plot.Visible?"=FALSE ("Plot.Visible")) -> (error out=w341:errorcluster)  [unwired: 1 in, 1 out]
                }
              }
              frame #1 {
                n190 = local read "S.3 SEL"() -> (w347:i32[])
                n191 = Array Size(array=w347) -> (size(s)=w346:i32)
                n192 = for {
                  N: w346 -> [_]
                  tunnel: w347 -> [w351] mode=indexing
                  tunnel: w348 -> [w354]
                  tunnel: w345 -> [w350] mode=indexing
                  n193 = Boolean To (0,1)(Boolean=w354) -> (0, 1=w353:i16)
                  n194 = property on="Graph S. 3" class="XYGraph （指定）"(error in=w350, "ActXScl"=w351, "YScale.Mapping Mode"=w353, "Plot.Visible?"=TRUE ("Plot.Visible")) -> (error out=→"error S3":errorcluster)  [unwired: 1 in, 1 out]
                }
              }
            }
            n195 = local read "log/linear 3"() -> (w337:bool)
          }
          frame #3 {
            n196 = flat-sequence {
              tunnel: w357 -> [w359]
              tunnel: [w358] -> w355
              tunnel: w356 -> [w367]
              tunnel: w355 -> [w364]
              frame #0 {
                n197 = for {
                  N: w359 -> [_]
                  tunnel: [w360] -> w358 mode=indexing
                  i -> [w363]
                  n198 = property on="Graph S. 4" class="XYGraph （指定）"(error in=errorcluster {"status"=FALSE, "code"=0, "source"=""} ("error in (no error)"), "Active Plot"=w363, "Plot.Visible?"=FALSE ("Plot.Visible")) -> (error out=w360:errorcluster)  [unwired: 1 in, 1 out]
                }
              }
              frame #1 {
                n199 = local read "S.4 SEL"() -> (w366:i32[])
                n200 = Array Size(array=w366) -> (size(s)=w365:i32)
                n201 = for {
                  N: w365 -> [_]
                  tunnel: w366 -> [w372] mode=indexing
                  tunnel: w367 -> [w373]
                  tunnel: w364 -> [w369] mode=indexing
                  n202 = Boolean To (0,1)(Boolean=w373) -> (0, 1=w370:i16)
                  n203 = property on="Graph S. 4" class="XYGraph （指定）"(error in=w369, "Active Plot"=w372, "Plot.Visible?"=TRUE ("Plot.Visible"), "YScale.Mapping Mode"=w370) -> (error out=→"error S4":errorcluster)  [unwired: 1 in, 1 out]
                }
              }
            }
            n204 = local read "log/linear 4"() -> (w356:bool)
          }
          frame #4 {
            n205 = flat-sequence {
              tunnel: w376 -> [w378]
              tunnel: [w377] -> w374
              tunnel: w375 -> [w386]
              tunnel: w374 -> [w383]
              frame #0 {
                n206 = for {
                  N: w378 -> [_]
                  tunnel: [w380] -> w377 mode=indexing
                  i -> [w382]
                  n207 = property on="Graph S. 5" class="XYGraph （指定）"(error in=errorcluster {"status"=FALSE, "code"=0, "source"=""} ("error in (no error)"), "Active Plot"=w382, "Plot.Visible?"=FALSE ("Plot.Visible")) -> (error out=w380:errorcluster)  [unwired: 1 in, 1 out]
                }
              }
              frame #1 {
                n208 = local read "S.5 SEL"() -> (w385:i32[])
                n209 = Array Size(array=w385) -> (size(s)=w384:i32)
                n210 = for {
                  N: w384 -> [_]
                  tunnel: w385 -> [w389] mode=indexing
                  tunnel: w386 -> [w392]
                  tunnel: w383 -> [w387] mode=indexing
                  n211 = Boolean To (0,1)(Boolean=w392) -> (0, 1=w391:i16)
                  n212 = property on="Graph S. 5" class="XYGraph （指定）"(error in=w387, "Active Plot"=w389, "YScale.Mapping Mode"=w391, "Plot.Visible?"=TRUE ("Plot.Visible")) -> (error out=→"error S5":errorcluster)  [unwired: 1 in, 1 out]
                }
              }
            }
            n213 = local read "log/linear 5"() -> (w375:bool)
          }
          frame #5 {
            n214 = flat-sequence {
              tunnel: w395 -> [w397]
              tunnel: [w396] -> w393
              tunnel: w394 -> [w405]
              tunnel: w393 -> [w402]
              frame #0 {
                n215 = for {
                  N: w397 -> [_]
                  tunnel: [w398] -> w396 mode=indexing
                  i -> [w401]
                  n216 = property on="Graph S. 6" class="XYGraph （指定）"(error in=errorcluster {"status"=FALSE, "code"=0, "source"=""} ("error in (no error)"), "Active Plot"=w401, "Plot.Visible?"=FALSE ("Plot.Visible")) -> (error out=w398:errorcluster)  [unwired: 1 in, 1 out]
                }
              }
              frame #1 {
                n217 = local read "S.6 SEL"() -> (w404:i32[])
                n218 = Array Size(array=w404) -> (size(s)=w403:i32)
                n219 = for {
                  N: w403 -> [_]
                  tunnel: w404 -> [w408] mode=indexing
                  tunnel: w405 -> [w411]
                  tunnel: w402 -> [w407] mode=indexing
                  n220 = Boolean To (0,1)(Boolean=w411) -> (0, 1=w409:i16)
                  n221 = property on="Graph S. 6" class="XYGraph （指定）"(error in=w407, "Active Plot"=w408, "YScale.Mapping Mode"=w409, "Plot.Visible?"=TRUE ("Plot.Visible")) -> (error out=→"error S6":errorcluster)  [unwired: 1 in, 1 out]
                }
              }
            }
            n222 = local read "log/linear 6"() -> (w394:bool)
          }
        }
        n223 = Index Array(array=w292, index (row) #1=0 ("index (row)"), index (row) #2=1 ("index (row)"), index (row) #3=2 ("index (row)"), index (row) #4=3 ("index (row)"), index (row) #5=4 ("disabled index (col)"), index (row) #6=5 ("index (col)"), index (row) #7=6 ("disabled index (row)"), index (row) #8=7 ("disabled index (row)"), index (row) #9=8 ("disabled index (row)")) -> (element #1=w254:dbl[], element #2=w259:dbl[], element #3=w263:dbl[], element #4=w256:dbl[], element #5=w255:dbl[], element #6=w253:dbl[], element #7=w240:dbl[], element #8=w239:dbl[], element #9=w238:dbl[])  [unwired: 9 in]
        n224 = stacked-sequence {
          tunnel: [w416 _ _ _ _ _ _ _ _] -> w273
          tunnel: [_ w425 _ _ _ _ _ _ _] -> w271
          tunnel: w270 -> [_ w423 w433 w442 w451 w460 w469 w478 w487]
          tunnel: w270 -> [w414 _ _ _ _ _ _ _ _]
          tunnel: [_ _ w431 _ _ _ _ _ _] -> w269
          tunnel: w259 -> [_ w421 _ _ _ _ _ _ _]
          tunnel: [_ _ _ w440 _ _ _ _ _] -> w266
          tunnel: [_ _ _ _ w449 _ _ _ _] -> w265
          tunnel: [_ _ _ _ _ w458 _ _ _] -> w264
          tunnel: w263 -> [_ _ w430 _ _ _ _ _ _]
          tunnel: [_ _ _ _ _ _ w467 _ _] -> w262
          tunnel: w256 -> [_ _ _ w439 _ _ _ _ _]
          tunnel: w255 -> [_ _ _ _ w448 _ _ _ _]
          tunnel: w254 -> [w412 _ _ _ _ _ _ _ _]
          tunnel: w253 -> [_ _ _ _ _ w457 _ _ _]
          tunnel: w240 -> [_ _ _ _ _ _ w466 _ _]
          tunnel: w239 -> [_ _ _ _ _ _ _ w472 _]
          tunnel: w238 -> [_ _ _ _ _ _ _ _ w481]
          tunnel: [_ _ _ _ _ _ _ w471 _] -> w237
          tunnel: [_ _ _ _ _ _ _ _ w480] -> w236
          frame #0 {
            # "P (4K)"
            n225 = Add Array Elements(numeric array=w412) -> (sum=w415:dbl)
            n226 = Divide(x=w415, y=w414) -> (x/y=w413:dbl)
            n227 = call "scaling_calculator.vi"("x1"=1.0, "y1"=0.0 ("x1"), "x"=w413, "x2"=3.0 ("x1"), "y2"=100000.0 ("x1")) -> ("y"=w416:dbl)  [unwired: 2 in]
          }
          frame #1 {
            # "LM"
            n228 = Add Array Elements(numeric array=w421) -> (sum=w424:dbl)
            n229 = Divide(x=w424, y=w423) -> (x/y=w422:dbl)
            n230 = call "scaling_calculator.vi"("x1"=0.0, "y1"=0.0 ("x1"), "x"=w422, "x2"=0.1 ("x1"), "y2"=100.0 ("x1")) -> ("y"=w425:dbl)  [unwired: 2 in]
          }
          frame #2 {
            # "Delta P He 4"
            n231 = Add Array Elements(numeric array=w430) -> (sum=w434:dbl)
            n232 = Divide(x=w434, y=w433) -> (x/y=w432:dbl)
            n233 = call "scaling_calculator.vi"("x1"=1.0, "y1"=0.0 ("x1"), "x"=w432, "x2"=5.0 ("x1"), "y2"=1000.0 ("x1")) -> ("y"=w431:dbl)  [unwired: 2 in]
          }
          frame #3 {
            # "Delta P He 3"
            n234 = Add Array Elements(numeric array=w439) -> (sum=w443:dbl)
            n235 = Divide(x=w443, y=w442) -> (x/y=w441:dbl)
            n236 = call "scaling_calculator.vi"("x1"=1.0, "y1"=0.0 ("x1"), "x"=w441, "x2"=5.0 ("x1"), "y2"=1000.0 ("x1")) -> ("y"=w440:dbl)  [unwired: 2 in]
          }
          frame #4 {
            # "FM He4"
            n237 = Add Array Elements(numeric array=w448) -> (sum=w452:dbl)
            n238 = Divide(x=w452, y=w451) -> (x/y=w450:dbl)
            n239 = call "scaling_calculator.vi"("x1"=0.0, "y1"=0.0 ("x1"), "x"=w450, "x2"=5.0 ("x1"), "y2"=500.0 ("x1")) -> ("y"=w449:dbl)  [unwired: 2 in]
          }
          frame #5 {
            # "FM He3"
            n240 = Add Array Elements(numeric array=w457) -> (sum=w461:dbl)
            n241 = Divide(x=w461, y=w460) -> (x/y=w459:dbl)
            n242 = call "scaling_calculator.vi"("x1"=0.0, "y1"=0.0 ("x1"), "x"=w459, "x2"=5.0 ("x1"), "y2"=200.0 ("x1")) -> ("y"=w458:dbl)  [unwired: 2 in]
          }
          frame #6 {
            # "BARATRON"
            n243 = Add Array Elements(numeric array=w466) -> (sum=w470:dbl)
            n244 = Divide(x=w470, y=w469) -> (x/y=w468:dbl)
            n245 = call "scaling_calculator_baratron.vi"("x"=w468) -> ("y (Pa)"=w467:dbl)  [unwired: 5 in, 1 out]
          }
          frame #7 {
            # "AI16 P 4He IN"
            n246 = Add Array Elements(numeric array=w472) -> (sum=w479:dbl)
            n247 = Divide(x=w479, y=w478) -> (x/y=w473:dbl)
            n248 = call "scaling_calculator.vi"("x1"=1.0, "y1"=0.0 ("x1"), "x"=w473, "x2"=5.0 ("x1"), "y2"=200000.0 ("x1")) -> ("y"=w471:dbl)  [unwired: 2 in]
          }
          frame #8 {
            # "AI17 P 3He OUT"
            n249 = Add Array Elements(numeric array=w481) -> (sum=w488:dbl)
            n250 = Divide(x=w488, y=w487) -> (x/y=w482:dbl)
            n251 = call "scaling_calculator.vi"("x1"=1.0, "y1"=0.0 ("x1"), "x"=w482, "x2"=5.0 ("x1"), "y2"=200000.0 ("x1")) -> ("y"=w480:dbl)  [unwired: 2 in]
          }
        }
        n252 = Build Array(w273, w271, w269, w266, w265, w264, w262, w237, w236) -> (w250:dbl[])
        "NI DAQ OUT" <- w250
        n253 = local read "current time"() -> (w230:timestamp)
        n254 = Build Array (concatenate)(w275, w250) -> (w233:dbl[][])
        n255 = Array To Cluster(array=w250) -> (cluster=w252:T8)
        n256 = To Double Precision Float(number=w230) -> (double precision float=w290:dbl)
        n257 = call "LV_UNIX.vi"("current time"=w230) -> ("date/time string"=w228:string, "UNIX time (s)"=w229:dbl)  [unwired: 9 in]
        n258 = Unbundle(w252) -> ("[0]"=w251:dbl, "[1]"=w249:dbl, "[2]"=w248:dbl, "[3]"=w247:dbl, "[4]"=w246:dbl, "[5]"=w245:dbl, "[6]"=w244:dbl, "[7]"=w235:dbl, "[8]"=w234:dbl)
        n259 = Index Array(array=w233, index (col) #1=0 ("disabled index (col)"), index (col) #2=1 ("disabled index (col)"), index (col) #3=2 ("disabled index (col)"), index (col) #4=3 ("disabled index (col)"), index (col) #5=4 ("index (col)"), index (col) #6=5 ("index (col)"), index (col) #7=6 ("index (col)"), index (col) #8=7 ("index (col)"), index (col) #9=8 ("index (col)")) -> (element #1=w286:dbl[], element #2=w284:dbl[], element #3=w282:dbl[], element #4=w280:dbl[], element #5=w277:dbl[], element #6=w276:dbl[], element #7=w260:dbl[], element #8=w221:dbl[], element #9=w220:dbl[])  [unwired: 9 in]
        n260 = Bundle(w232, w220) -> (w212:cluster{dbl[], dbl[]})  [unwired: 1 in]
        n261 = Bundle(w232, w286) -> (w225:cluster{dbl[], dbl[]})  [unwired: 1 in]
        n262 = Bundle(w232, w284) -> (w224:cluster{dbl[], dbl[]})  [unwired: 1 in]
        n263 = Bundle(w232, w282) -> (w219:cluster{dbl[], dbl[]})  [unwired: 1 in]
        n264 = Bundle(w232, w280) -> (w218:cluster{dbl[], dbl[]})  [unwired: 1 in]
        n265 = Bundle(w232, w277) -> (w217:cluster{dbl[], dbl[]})  [unwired: 1 in]
        n266 = Bundle(w232, w276) -> (w216:cluster{dbl[], dbl[]})  [unwired: 1 in]
        n267 = Bundle(w232, w260) -> (w214:cluster{dbl[], dbl[]})  [unwired: 1 in]
        n268 = Bundle(w232, w221) -> (w215:cluster{dbl[], dbl[]})  [unwired: 1 in]
        n269 = local read "error out\n(file creation)"() -> (w289:errorcluster)
        n270 = local read "ref DAQ"() -> (w288:refnum<file>)
        n271 = local read "Cycle #"() -> (w227:i32)
        n272 = Format Into String(format string="%d,%s,%10.4f,%10.4f,%5.6f,%5.6f,%5.6f,%5.6f,%5.6f,%5.6f,%5.6f,%5.6f,%5.6f\\n", initial string=w288, error in=w289, w227, w228, w229, w290, w251, w249, w248, w247, w246, w245, w244, w235, w234) -> (error out=→"error out \n(record DAQ)":errorcluster)  [unwired: 1 out]
        n273 = Build Array(w225, w224, w219, w218, w217, w216, w215, w214, w212) -> (→"Graph S. 1" →"Graph S. 2" →"Graph S. 3" →"Graph S. 4" →"Graph S. 5" →"Graph S. 6":cluster{dbl[], dbl[]}[])
      }
      frame #1 {
        n274 = local read "error out \n(DAQ IN)"() -> (w490:errorcluster)
        n275 = local read "DAQ OUT ON?"() -> (w492:bool)
        n276 = case shown="TRUE" w492 {
          tunnel: w493 -> [w495 w500]
          tunnel: [w495 w499] -> w491
          tunnel: w490 -> [w494 w497]
          tunnel: [w494 w496] -> w489
          frame False {
          }
          frame True {
            n277 = call <vilib>:"DAQmx Write (Analog 1D DBL 1Chan NSamp).vi"("task/channels in"=w500, "data"="DAQ OUT SET Volt", "timeout"=100.0, "error in"=w497) -> ("task out"=w499:refnum<k21>, "number of samples written per channel"=→"DAQ OUT \nsample #":u32, "error out"=w496:errorcluster)  [unwired: 9 in]
          }
        }
        "error out\n(DAQ OUT)" <- w489
      }
    }
    "Cycle #" <- w205
  }
  n278 = call <vilib>:"DAQmx Stop Task.vi"("task/channels in"=w11, "error in"=w9) -> ("task out"=w13:refnum<k21>, "error out"=w12:errorcluster)  [unwired: 12 in]
  n279 = call <vilib>:"DAQmx Clear Task.vi"("task in"=w13, "error in"=w12) -> ("error out"=w15:errorcluster)  [unwired: 13 in]
  n280 = call <vilib>:"DAQmx Stop Task.vi"("task/channels in"=w10, "error in"=w15) -> ("task out"=w17:refnum<k21>, "error out"=w14:errorcluster)  [unwired: 12 in]
  n281 = call <vilib>:"DAQmx Clear Task.vi"("task in"=w17, "error in"=w14) -> ("error out"=→"error out DAQ Final state":errorcluster)  [unwired: 13 in]
